vi "UHR-Fleezers Control (fpga) - 11.4b.vi"() -> ()   [LabVIEW 2012]
doc: "UHR-Fleezers Instrument Control Code (fpga)"
uses:
  <vilib>/Platform/TimedLoop/XDataNode/timing_clust.ctl
  <vilib>/Platform/TimedLoop/XDataNode/nitl_modes.ctl
  <vilib>/Platform/TimedLoop/XDataNode/wakeup.ctl
  <vilib>/rvi/eio/common/nirviEmuTemplateMethod_errors.vi
  <vilib>/rvi/interface/RandomDataEmulation/nirviRandomDataFPGAFIFO.vi
  <vilib>/rvi/interface/RandomDataEmulation/niFpgaRandomDataHandleErrors.vi
  <vilib>/rvi/Emulation/niFpgaSctlEmulationGetInTimedLoop.vi
  <vilib>/rvi/Emulation/niFpgaSctlEmulationGlobalWrite.vi
  <vilib>/rvi/Emulation/niFpgaSctlEmulationRegisterWithScheduler.vi
  <vilib>/rvi/Emulation/niFpgaSctlEmulationScheduler.vi
  <vilib>/Platform/TimedLoop/XDataNode/XDataNode.xnode
  <vilib>/eio/EIOMethodNode/EIOMethodNode.xnode
  <vilib>/eio/EIONode/EIONode.xnode
  <vilib>/rvi/DataTransferAndStorage/Container/XNode/niFpgaContainer.xnode
  <vilib>/rvi/interface/RandomDataEmulation/nirviRandomDataFpgaReadWriteTemplate.vi
  <vilib>/addons/control/pid/fpga.llb/XNode/niFpgaPID.xnode
  <vilib>/Platform/TimedLoop/XDataNode/XDNodeRunTimeDep.lvlib
panel:
  in  "Tab Control":T1(tab)=enum."Force FB"
  in  "Set 3":bool
  in  "Set 2":bool=TRUE
  in  "Set 1":bool=TRUE
  in  "Trap Pos to FIFO":bool
  in  "N of AI1 Int Acq Sets":i16=2 min=1 max=3 step=1
  out "AI Late Counter":u8
  in  "ai count":u16=400
  in  "+ phase":bool
  in  "Phase count adjustment":i16
  out "Relative phase":i16
  in  "AI to FIFO":bool
  out "BD1 Frequency Out 1":u64
  out "BD1 Frequency Out 2":u64
  out "Trap Pos FIFO Timeout":u16
  out "Trap AI FIFO Timeout":u16
  in  "Trap FIFO Set Timeout":i32
  in  "Tab Control 2":T2(tab)
  in  "RD":bool
  in  "FB1 output high":i16=3000
  in  "FB1 output low":i16
  in  "D1":i16
  in  "I1":i16=5
  in  "P1":i16=10
  in  "Swap F1 and F2":bool
  in  "Cont. Scan":bool
  in  "Abort scan":bool
  in  "Cycles per step":u64
  in  "Scan BD":bool
  in  "Number of scans":u16
  in  "Scan steps":u64
  in  "Scan freq.  increment":i64
  out "Scanning":bool
  in  "Start scan":bool
  in  "OSK Bd 1":bool
  in  "Reset Bd 1":bool
  in  "PMODE":bool
  in  "Direct RF Box \nCommunication":bool
  in  "Data BD 2":u8 format="%08b"
  in  "Data BD 1":u8 format="%08b"
  in  "Address":u8 format="%02x"
  in  "Update Data":bool
  in  "FPGA Controls\n RF Box":bool
  in  "Number Interlace Cycles":u8=2 min=1 max=3
  in  "Interlace Off Parameters":u8=1 min=1 max=3
  in  "Interlace ON/OFF":bool
  out "DIO Relative phase":i16
  in  "Phase count adjustment (DIO)":i16
  in  "+ phase (DIO)":bool
  out "DIO Late Counter":u8
  in  "DIO count 1 (ticks)":u16=400
  in  "DIO count 2 (ticks)":u16=400
  in  "DIO count 3 (ticks)":u16=400
  out "AI2 Y Sum Set 2":i16
  out "AI2 Y Sum Set 1":i16
  in  "FB Setpoint Set 1":i16 min=0 step=1
  in  "FB Reset Set 1":bool
  in  "FB On/Off Set 1":bool
  in  "FB Reset Set 2":bool
  in  "FB On/Off Set 2":bool
  in  "FB Setpoint Set 2":i16 min=0 step=1
  out "Scan I":u64
  in  "Amp switch delay":u8=5
  in  "BD 2 Amplitude 1":u16
  in  "BD 1 Amplitude 1":u16
  in  "BD 2 Frequency 1":u64
  in  "BD 1 Frequency 1":u64
  in  "BD 2 Amplitude 2":u16
  in  "BD 1 Amplitude 2":u16
  in  "BD 2 Frequency 2":u64
  in  "BD 1 Frequency 2":u64
  in  "BD 2 Amplitude 3":u16
  in  "BD 1 Amplitude 3":u16
  in  "BD 2 Frequency 3":u64
  in  "BD 1 Frequency 3":u64
  in  "BD 1 Delay (ticks)":u8
  in  "BD 2 Delay (Ticks)":u8 caption="Count(Ticks)"
  in  "FB2 output high":fxp<+/-,16,1>=0.999969482421875
  in  "FB2 output low":fxp<+/-,16,1>=-1.0
  in  "P2":fxp<+/-,16,8> format="%.11g"
  in  "I2":fxp<+/-,16,8>=10.0 format="%.11g"
  in  "D2":fxp<+/-,16,8> format="%.11g"
  in  "Negate Diff?":bool
  in  "Diff FB Measurement?":bool
  in  "FB Trig Integrate":u32=1
  out "TTrig?":bool
  in  "TTrig Negate Pos":bool=TRUE
  out "Trap Pos FB Int Signal":fxp<+/-,24,9> format="%.18g"
  out "Trap Pos FB Int-Norm Signal":fxp<+/-,16,1> format="%.16g"
  in  "FPGA TTrig Thresh":i64
  in  "FPGA Trap Trig":bool
  out "Trap Pos FB Action":i64
  in  "Trap Pos. FB Offset Factor":i64
  in  "Trap Pos. FB Mult Factor":i64=2
  in  "Trap Pos. FB Reset":bool
  in  "Trap Pos FB Monitor T1 or T2":bool
  in  "AI1 X Scale":u16
  in  "Trap Pos FB Int Count":u16=100
  in  "Trap Pos FB Negate Action":bool
  out "AI1 X Set 2":fxp<+/-,16,1>
  out "AI1 X Set 1":fxp<+/-,16,1>
  in  "Trap Pos. FB SP":fxp<+/-,16,1>
  in  "Force feedback":bool
  out "TTrig Sig":i64
  out "TTrig Fin Thresh":i64
  in  "1D or 2D Scan?":bool
  in  "Abort scan (MCL)":bool
  in  "MCL Scan Axis":bool
  in  "Cont. Scan (MCL)":bool
  out "Scan I (MCL)":u64
  in  "Number of scans (MCL)":u16
  out "Scanning MCL":bool
  in  "Scan steps (MCL)":u64
  in  "Cycles per step (MCL)":u64
  in  "Scan freq.  increment (MCL)":i16
  in  "Start scan (MCL)":bool
  in  "AO2":i16
  in  "AO1":i16
  out "MCL Late Counter":u8
  in  "MCL count":u32=800
  out "MCL Relative Phase":i16
  in  "Phase count adjustment (MCL)":i16
  in  "+ phase (MCL)":bool
  out "APD3 out state":bool
  in  "APD Gate Operating Mode":u8 max=2 step=1
  in  "Invert APD Gate":bool
  in  "APD Gate OFF Count":u16=100
  in  "APD Gate ON Count":u16=300
  out "APD 1 Gate Late Counter":u8
  out "APD 1 Gate Relative Phase":i16
  in  "Phase count adjustment (APD 1 Gate)":i16
  in  "+ phase (APD 1 Gate)":bool
  out "APD 2 Counts 0":u32
  out "APD 2 Counts 1":u32
  out "APD 1 Counts 0":u32
  out "APD 1 Counts 1":u32
  out "APD1 out state":bool
  in  "APD AO scale factor":i16=1
  in  "APD to FIFO":bool
  in  "APD Acq Rate Count":u32=20000000
  out "APD Acq Late Counter":u8
  out "APD Acq Relative Phase":i16
  in  "Phase Count Adjustment (APD Acq)":i16
  in  "+ phase (APD Acq)":bool
  in  "Phase count adjustment (APD 2 Gate)":i16
  out "APD 2 Gate Late Counter":u8
  out "APD 2 Gate Relative Phase":i16
  in  "+ phase (APD 2 Gate)":bool
  out "APD2 out state":bool
  out "APD 3 Counts 0":u32
  out "APD 3 Counts 1":u32
  out "APD 3 Gate Late Counter":u8
  in  "Phase count adjustment (APD 3 Gate)":i16
  out "APD 3 Gate Relative Phase":i16
  in  "+ phase (APD 3 Gate)":bool
  in  "D3":i16
  in  "I3":i16=5
  in  "P3":i16=10
  in  "Green Filter Flipper":bool
  in  "Green FB Count":u16=1200
  out "Green Late Counter":u8
  out "Green FB Relative Phase":i16
  in  "Phase count adjustment (Green FB)":i16=10
  in  "+ phase (Green FB)":bool
  out "Green FB Sum":i16
  in  "Green int current ON count adj":u16=150
  in  "Current Out":u16=30000
  in  "Green FB On/Off":bool
  in  "Green FB Setpoint":i16=250 min=0 step=1
  in  "Green FB Reset":bool
  in  "Operating Mode 2":u8=2 max=2 step=1
  in  "Invert GI 2":bool
  in  "Green interlace OFF count 2":u16=900
  in  "Green interlace ON count 2":u16=300
  out "GI Late Counter 2":u8
  out "GI Relative phase 2":i16
  in  "Phase count adjustment (GI) 2":i16=20
  in  "+ phase (GI) 2":bool
  in  "Green interlace OFF count":u16=100
  out "GI Relative phase":i16
  in  "Phase count adjustment (GI)":i16
  in  "+ phase (GI)":bool
  in  "Green interlace ON count":u16=300
  out "GI Late Counter":u8
  in  "Invert GI":bool
  in  "Operating Mode":u8 max=2 step=1
  in  "+ phase (RI)":bool
  out "RI Relative phase":i16
  out "RI Late Counter":u8
  in  "Red interlace ON count":u16=300
  in  "Red interlace OFF count":u16=100
  in  "Invert RI":bool
  in  "Red Laser Operating Mode":u8 max=2 step=1
  in  "Phase count adjustment (RI)":i16
  out "Red FB Intensity":i16
  in  "RI Current Out":u16=30000
  in  "Red FB On/Off":bool
  in  "D4":i16
  in  "I4":i16=5
  in  "P4":i16=10
  in  "Red FB Setpoint":i16=250 min=0 step=1
  in  "Red FB Reset":bool
  in  "RI Operating Mode 2":u8=2 max=2 step=1
  in  "Invert RI 2":bool
  in  "Phase count adjustment (BI AO)":i16=20
  in  "Blue current ON count adj (AO)":u16=150
  in  "BI Current Out":i16=30000
  in  "Blue FB On/Off":bool
  in  "D5":i16
  in  "I5":i16=5
  in  "P5":i16=10
  in  "Blue FB Setpoint":i16=250 min=0 step=1
  in  "Blue FB Reset":bool
  in  "BI Operating Mode (AO)":u8=2 max=2 step=1
  in  "Invert BI (AO)":bool
  in  "Blue OFF count (AO)":u16=900
  in  "Blue ON count (AO)":u16=300
  out "BI Late Counter (AO)":u8
  out "BI Relative phase (AO)":i16
  in  "+ phase (BI AO)":bool
  in  "Phase count adjustment (BI D)":i16
  in  "Blue Laser Operating Mode (D)":u8 max=2 step=1
  in  "Invert BI (D)":bool
  in  "Blue interlace OFF count (D)":u16=100
  in  "Blue interlace ON count (D)":u16=300
  out "Blue Late Counter (D)":u8
  out "BI Relative phase (D)":i16
  in  "+ phase (BI D)":bool
  out "Blue Intensity":i16
  # "Only one of these can be on\nat a time:"
  # "Raster Scan AOD"
  # "1 (X)"
  # "2 (Y)"
  # "IR Intensity Feedback (RF BD 1)"
  # "FB Gains Set 1"
  # "FB output range 1"
  # "FB Triggering Excitation Laser"
  # "Trap Pos. FB Gains"
  # "Trap Pos. FB Range"
  # "AO1 (Y)"
  # "2D"
  # "1D"
  # "AO2 (X)"
  # "APD AO for aligning"
  # "Detection Loop"
  # "Green fluorescent laser digital gate interlacing loop"
  # "0 Forced ON\n1 Forced OFF\n2 Interlacing"
  # "Green FB Gains"
  # "Red fluorescent laser digital gate interlacing loop"
  # "Detection Loop"
  # "0 Forced ON\n1 Forced OFF\n2 Interlacing"
  # "Analog/FB Control Loop\n(Disabled)"
  # "Digital Control Loop"
  # "Blue laser intensity reading"
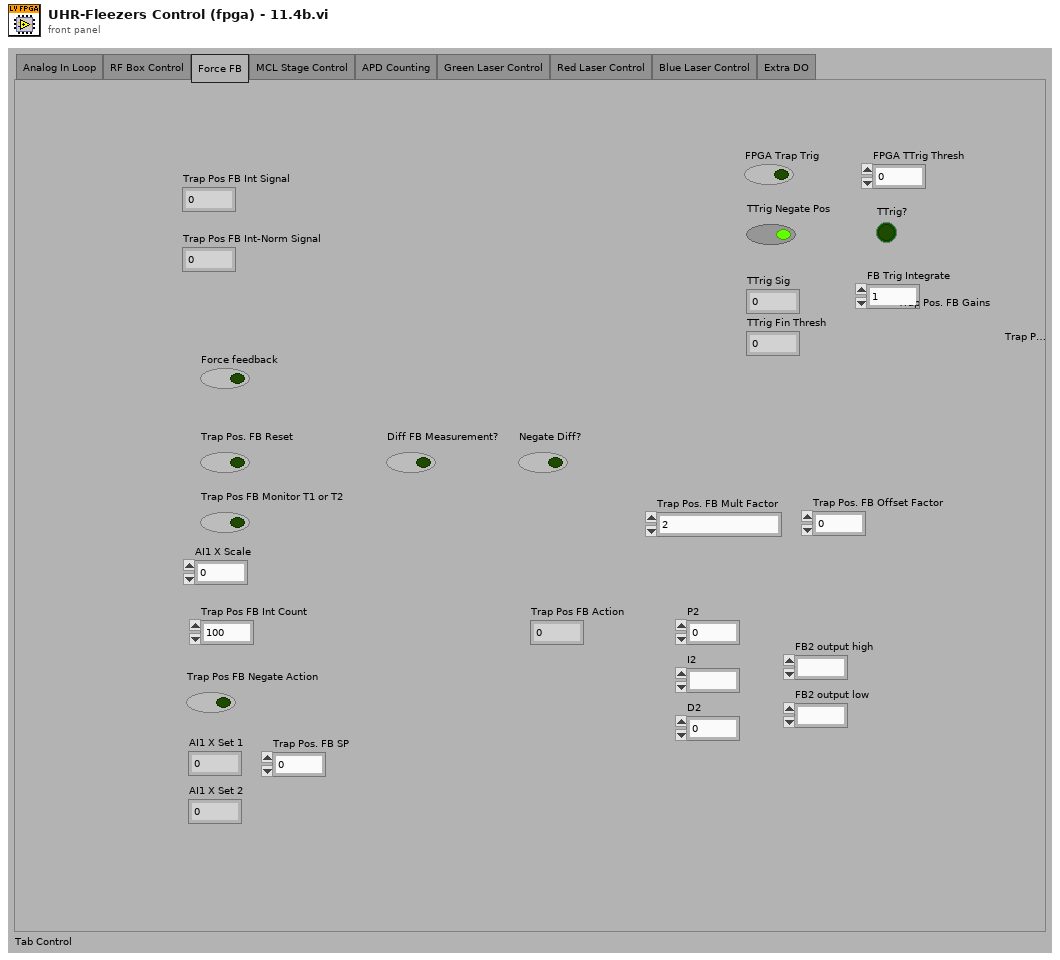
[diagram p1: front panel]
types:
  T1 = enum32{"Analog In Loop", "RF Box Control", "Force FB", "MCL Stage Control", "APD Counting", "Green Laser Control", "Red Laser Control", "Blue Laser Control", "Extra DO"}
  T2 = enum32{"Controls", "Interlacing Frequency and Amplitude Values"}
  T3 = typedef "XDNodeRunTimeDep.lvlib/timing_clust.ctl" = cluster{"Expected End [f-1]":u64, "Actual End [f-1]":u64, "Finished Late? [f-1]":bool, "Expected End [i-1]":u64, "Actual End [i-1]":u64, "Finished Late? [i-1]":bool, "Expected Start [i]":u64, "Actual Start [i]":u64, "Expected Start [f]":u64, "Actual Start [f]":u64, "Source Name":string, "Structure Name":string, "Period":i64, "Deadline":i64, "Offset":i64, "Start":i64, "Priority":i32, "Timeout":i32, "Mode":T4, "Wakeup Reason":T5, "Error":errorcluster, "Source Type":string, "Secondary Source Type":string, "Global End Time":u64, "Global Start Time":u64, "Frame Duration":u64, "Iteration Duration":u64, "Assigned CPU":i32, "I/O Scan Engine Mode":u32}
  T4 = typedef "XDNodeRunTimeDep.lvlib/nitl_modes.ctl" = enum32{"No Change", "Process missed periods, maintain original phase", "Discard missed periods, maintain original phase", "Process missed periods, ignore original phase", "Discard missed periods, ignore original phase"}
  T5 = typedef "XDNodeRunTimeDep.lvlib/wakeup.ctl" = enum32{"Normal", "Aborted", "Asynchronous wakeup", "Timing source error", "Timed loop error", "Timeout"}
  T6 = cluster{"proportional gain (Kc)":i16, "integral gain (Kc*Ts/Ti)":i16, "derivative gain (Kc*Td/Ts)":i16}
  T7 = cluster{"FB1 output high":i16, "FB1 output low":i16}
  T8 = cluster{"P2":fxp<+/-,16,8>, "I2":fxp<+/-,16,8>, "D2":fxp<+/-,16,8>}
  T9 = cluster{"FB2 output high":fxp<+/-,16,1>, "FB2 output low":fxp<+/-,16,1>}
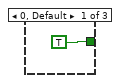
[diagram p3: hidden frame]
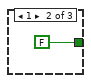
[diagram p4: hidden frame]
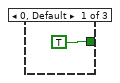
[diagram p5: hidden frame]
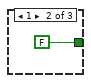
[diagram p6: hidden frame]
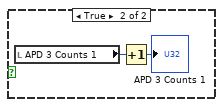
[diagram p7: hidden frame]
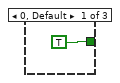
[diagram p8: hidden frame]
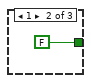
[diagram p9: hidden frame]
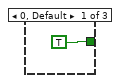
[diagram p10: hidden frame]
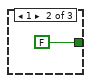
[diagram p11: hidden frame]
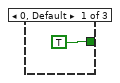
[diagram p12: hidden frame]
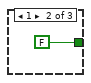
[diagram p13: hidden frame]
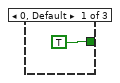
[diagram p14: hidden frame]
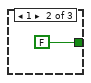
[diagram p15: hidden frame]
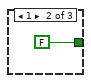
[diagram p18: hidden frame]
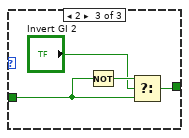
[diagram p19: hidden frame]
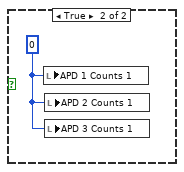
[diagram p20: hidden frame]
diagram:
  w3 = u16 0
  w5 = FALSE
  w2 = FALSE
  # "timing array current index"
  # "timing array"
  # "timing counter (phase adjusted here)"
  # "late counter"
  n1 = flat-sequence "FPGA initialization to do before running any of the loops" {
    tunnel: [u16 0 ("DIO count 3 (ticks)")] -> w1
    tunnel: [w13] -> _
    frame #0 {
      w12 = FALSE ("Enable")
      # "BD 2 (Y)"
      # "BD 1 (X)"
      # "Start up expansion chassis early\nto avoid delays later"
      # "This pin controls udclk on the RF boards.\nWhen initially configuring the boards, this pin needs to be\nconfigured as a high impedance input.  Later it will be switched\nto an output."
      # "Initial setting of DIO data and \naddress to low (before reset).  \nThis needs to happen before the other\ncontrol method loops execute."
      n2 = xnode "FPGA I/O Node"("Chassis2/Mod4/AO0"=u16 0) -> ("Chassis2/Mod1/AI0"=w13:i16)  [unwired: 2 in, 2 out]
      n3 = xnode "FPGA I/O Method Node"("Enable"=w12) -> ()  [unwired: 1 in, 1 out]
      n4 = xnode "FPGA I/O Method Node"("Enable"=w12) -> ()  [unwired: 1 in, 1 out]
      n5 = xnode "FPGA I/O Node"("Connector1/DIO0"=FALSE, "Connector1/DIO1"=FALSE, "Connector1/DIO2"=FALSE, "Connector1/DIO3"=FALSE, "Connector1/DIO4"=FALSE, "Connector1/DIO5"=FALSE, "Connector1/DIO6"=FALSE, "Connector1/DIO7"=FALSE, "Connector1/DIO8"=FALSE, "Connector1/DIO9"=FALSE, "Connector1/DIO10"=FALSE, "Connector1/DIO11"=FALSE, "Connector1/DIO12"=FALSE, "Connector1/DIO13"=FALSE, "Connector1/DIO15"=FALSE, "Connector1/DIO20"=FALSE, "Connector1/DIO21"=FALSE, "Connector1/DIO22"=FALSE, "Connector1/DIO23"=FALSE, "Connector1/DIO24"=FALSE, "Connector1/DIO25"=FALSE, "Connector1/DIO26"=FALSE, "Connector1/DIO27"=FALSE, "Connector1/DIO14"=FALSE) -> ()  [unwired: 24 in, 24 out]
    }
  }
  n6 = local read "AO1"() -> (w10:i16)
  n7 = local read "AO2"() -> (w9:i16)
  n8 = node-c288() -> (w8:T3)  [unwired: 1 in]
  n9 = timed-loop "RF box board DIO control: control bits" {
    timing: w8 -> [_]
    timing-out: [_] -> w7
    tunnel: [w42] -> _
    tunnel: w1 -> [w42]
    stop <- FALSE stop-if-true
    n10 = xnode "FPGA I/O Node"("Connector1/DIO16"="RD", "Connector1/DIO17"="PMODE", "Connector1/DIO18"="OSK Bd 1", "Connector1/DIO19"="Reset Bd 1", "Connector0/DIO3"="Green Filter Flipper") -> ()  [unwired: 5 in, 5 out]
  }
  n11 = while "RF box board DIO control: parallel communication" {
    shift-right: [w55] -> _
    shift-left: w1 -> [w54]
    shift-right: [w53] -> _
    shift-left: FALSE ("Swap F1 and F2") -> [w52]
    stop <- FALSE stop-if-true
    n12 = flat-sequence {
      tunnel: w52 -> [w59]
      tunnel: w54 -> [w57]
      tunnel: [w59] -> w51
      tunnel: [w58] -> w50
      tunnel: [w57] -> w49
      tunnel: [w65] -> w55
      tunnel: [w64] -> w53
      tunnel: w51 -> [w63]
      tunnel: w50 -> [w61]
      tunnel: w49 -> [w60]
      frame #0 {
        n13 = call "Loop Timer"("Count(Ticks)"=w57) -> ("Tick Count(Ticks)"=w58:u16)
      }
      frame #1 {
        n14 = flat-sequence {
          tunnel: ["FPGA Controls\n RF Box"] -> w62
          tunnel: w63 -> [w66]
          tunnel: [w116] -> w65
          tunnel: [w129] -> w64
          tunnel: w62 -> [w128]
          tunnel: w61 -> [w122]
          tunnel: w60 -> [w119]
          frame #0 {
            n15 = case shown="True" "FPGA Controls\n RF Box" {
              tunnel: w66 -> [_ w68]
              frame False {
              }
              frame True {
                n16 = flat-sequence {
                  tunnel: w68 -> [w78]
                  frame #0 {
                    n17 = First Call?() -> (First Call?: T/F=w69:bool)
                    n18 = case shown="True" w69 {
                      frame False {
                      }
                      frame True {
                        # "BD 2"
                        # "BD 1"
                        # "If first time data updated, be sure to set WR high and UDCLK low\nbefore setting data and address bits."
                        n19 = xnode "FPGA I/O Method Node"("Enable"=TRUE) -> ("FPGA I/O Out"=w71:refnum<k21>)  [unwired: 1 in]
                        n20 = xnode "FPGA I/O Method Node"("Enable"=TRUE) -> ("FPGA I/O Out"=w74:refnum<k21>)  [unwired: 1 in]
                        n21 = xnode "FPGA I/O Node"("Connector1/DIO15"=TRUE) -> ()  [unwired: 1 in, 1 out]
                        n22 = xnode "FPGA I/O Node"("I/O Item"=FALSE ("Connector1/DIO30"), "FPGA I/O In"=w71) -> ()  [unwired: 1 out]
                        n23 = xnode "FPGA I/O Node"("I/O Item"=FALSE ("Connector1/DIO30"), "FPGA I/O In"=w74) -> ()  [unwired: 1 out]
                      }
                    }
                  }
                  frame #1 {
                    n24 = flat-sequence "BD 1 (X)" {
                      tunnel: w78 -> [w85]
                      tunnel: "Amp switch delay" -> [w86]
                      frame #0 {
                        n25 = call "Wait6"("Count(Ticks)"="BD 1 Delay (ticks)") -> ()  [unwired: 1 out]
                      }
                      frame #1 {
                        # "switch frequency"
                        n26 = xnode "FPGA I/O Node"("Connector1/DIO36"=w85) -> ()  [unwired: 1 in, 1 out]
                      }
                      frame #2 {
                        # "~5 ticks is usual"
                        n27 = call "Wait4"("Count(Ticks)"=w86) -> ()  [unwired: 1 out]
                      }
                      frame #3 {
                        # "this switches amplitude"
                        # "switch amplitude"
                        # "send udclk high"
                        n28 = xnode "FPGA I/O Node"("Connector1/DIO30"=TRUE ("Connector1/DIO15")) -> ()  [unwired: 1 in, 1 out]
                      }
                      frame #4 {
                        # "reset to be ready for next\ncycle"
                        # "send udclk low"
                        n29 = xnode "FPGA I/O Node"("Connector1/DIO30"=FALSE ("Connector1/DIO15")) -> ()  [unwired: 1 in, 1 out]
                      }
                    }
                    n30 = flat-sequence "BD 2 (Y)" {
                      tunnel: w78 -> [w80]
                      tunnel: "Amp switch delay" -> [w81]
                      frame #0 {
                        n31 = call "Wait7"("Count(Ticks)"="BD 2 Delay (Ticks)") -> ()  [unwired: 1 out]
                      }
                      frame #1 {
                        # "switch frequency"
                        n32 = xnode "FPGA I/O Node"("Connector1/DIO37"=w80) -> ()  [unwired: 1 in, 1 out]
                      }
                      frame #2 {
                        # "~5 ticks is usual"
                        n33 = call "Wait5"("Count(Ticks)"=w81) -> ()  [unwired: 1 out]
                      }
                      frame #3 {
                        # "this switches amplitude"
                        # "switch amplitude"
                        # "send udclk high"
                        n34 = xnode "FPGA I/O Node"("Connector1/DIO29"=TRUE ("Connector1/DIO15")) -> ()  [unwired: 1 in, 1 out]
                      }
                      frame #4 {
                        # "reset to be ready for next\ncycle"
                        # "send udclk low"
                        n35 = xnode "FPGA I/O Node"("Connector1/DIO29"=FALSE ("Connector1/DIO15")) -> ()  [unwired: 1 in, 1 out]
                      }
                    }
                  }
                }
              }
            }
          }
          frame #1 {
            # "This is the prior cycle's on time"
            # "increment timing\nindex, reset to 0 if \nend of matrix"
            # "Reset to begginning (1) when number of cycles reached."
            # "timing index"
            # "build byte stacks for writing data\n(must correspond to addresses array constant)"
            # "Timing housekeeping"
            # "Adjust phase if late\n(maintains constant phase relationship between cycles)"
            n36 = Bundle("FB1 output high"="FB1 output high", "FB1 output low"="FB1 output low") -> (w89:T7)  [unwired: 1 in]
            n37 = Bundle("P1"="P1", "I1"="I1", "D1"="D1") -> (w90:cluster{"P1":i16, "I1":i16, "D1":i16})  [unwired: 1 in]
            n38 = feedback #1(u8 0 ("t")) -> (w125:u8)
            n39 = Increment(x=w125) -> (x+1=w169:u8)
            n40 = Increment(x="Number Interlace Cycles") -> (x+1=w164:u8)
            n41 = Equal?(x=w169, y=w164) -> (x = y?=w171:bool)
            n42 = Select(t=u8 1, s=w171, f=w169) -> (s? t:f=w124:u8)
            n43 = feedback-in #1(w124) -> ()
            n44 = Increment(x=w124) -> (x+1=w166:u8)
            n45 = Equal?(x=w166, y=w164) -> (x = y?=w167:bool)
            n46 = Select(t=u8 1, s=w167, f=w166) -> (s? t:f=w163:u8)
            n47 = Select(t=w163, s="Interlace ON/OFF", f="Interlace Off Parameters") -> (s? t:f=w147:u8)
            n48 = case shown="1, Default" w147 {
              tunnel: [w243 "BD 1 Frequency 2" "BD 1 Frequency 3"] -> w159
              tunnel: [w242 "BD 2 Frequency 2" "BD 2 Frequency 3"] -> w148
              tunnel: ["BD 2 Amplitude 1" "BD 2 Amplitude 2" "BD 2 Amplitude 3"] -> w104
              tunnel: [w231 w402 "BD 1 Amplitude 3"] -> w107
              tunnel: w90 -> [w205 w399 _]
              tunnel: w89 -> [w206 w398 _]
              frame 1, Default {
                w222 = fxp<+/-,24,9> 0.0 ("AI1 X Set 2")
                w215 = u16 0
                w238 = u64 0 ("f")
                # "This signal integration happens no matter what\nso that correct setpoints can be chosen before \nturning on the FB."
                # "Trap 1"
                n49 = local read "AI1 X Set 2"() -> (w218:fxp<+/-,16,1>)
                n50 = local read "AI1 X Set 1"() -> (w219:fxp<+/-,16,1>)
                n51 = local read "Scanning"() -> (w244:bool)
                n52 = Or(x=w244, y="Start scan") -> (x .or. y?=w236:bool)
                n53 = case shown="False" "Diff FB Measurement?" {
                  tunnel: w218 -> [w252 w261]
                  tunnel: w219 -> [w251 w262]
                  tunnel: [w249 w253] -> w220
                  frame False {
                    n54 = Select(t=w251, s="Trap Pos FB Monitor T1 or T2", f=w252) -> (s? t:f=w249:fxp<+/-,16,1>)
                  }
                  frame True {
                    n55 = Subtract(x=w262, y=w261) -> (x-y=w254:fxp<+/-,17,2>)
                    n56 = Not(x="Negate Diff?") -> (.not. x?=w260:bool)
                    n57 = Boolean To (0,1)(Boolean="Negate Diff?") -> (0, 1=w258:i16)
                    n58 = Boolean To (0,1)(Boolean=w260) -> (0, 1=w259:i16)
                    n59 = Negate(x=w258) -> (-x=w257:i16)
                    n60 = Add(x=w257, y=w259) -> (x+y=w255:i16)
                    n61 = Multiply(x=w255, y=w254) -> (x*y=w253:fxp<+/-,32,17>)
                  }
                }
                n62 = Not(x="Abort scan") -> (.not. x?=w234:bool)
                n63 = And(x=w234, y=w236) -> (x .and. y?=w233:bool)
                n64 = case "For raster scanning" shown="True" w233 {
                  tunnel: [u64 0 w388] -> w239
                  tunnel: "Start scan" -> [_ w373]
                  frame False {
                    n65 = local write "Scanning"(FALSE ("scanning")) -> ()
                  }
                  frame True {
                    w357 = i64 0
                    w356 = u64 0
                    # "scan incr."
                    # "freq. incr. mult."
                    # "count steps"
                    # "count number of cycles"
                    n66 = feedback #2(w356) -> (w385:u64)
                    n67 = Select(t=w356, s=w373, f=w385) -> (s? t:f=w387:u64)
                    n68 = Increment(x=w387) -> (x+1=w384:u64)
                    n69 = Greater?(x="Cycles per step", y=w384) -> (0:w366:bool)
                    n70 = Select(t=w384, s=w366, f=w356) -> (s? t:f=w383:u64)
                    n71 = feedback-in #2(w383) -> ()
                    n72 = feedback #3(w356) -> (w382:u64)
                    n73 = Select(t=w356, s=w373, f=w382) -> (s? t:f=w377:u64)
                    n74 = Increment(x=w377) -> (x+1=w381:u64)
                    n75 = Add(x="Scan steps", y="Scan steps") -> (x+y=w380:u64)
                    n76 = Select(t=w377, s=w366, f=w381) -> (s? t:f=w361:u64)
                    n77 = Greater?(x=w380, y=w361) -> (0:w360:bool)
                    n78 = Select(t=w361, s=w360, f=w356) -> (s? t:f=w378:u64)
                    n79 = feedback-in #3(w378) -> ()
                    n80 = Equal?(x="Scan steps", y=w361) -> (x = y?=w365:bool)
                    n81 = Greater?(x="Scan steps", y=w377) -> (0:w376:bool)
                    n82 = feedback #4(w357) -> (w379:i64)
                    n83 = Select(t=w357, s=w373, f=w379) -> (s? t:f=w363:i64)
                    n84 = Increment(x=w363) -> (x+1=w375:i64)
                    n85 = Decrement(x=w363) -> (x-1=w374:i64)
                    n86 = Select(t=w375, s=w376, f=w374) -> (s? t:f=w364:i64)
                    n87 = Select(t=w363, s=w365, f=w364) -> (s? t:f=w362:i64)
                    n88 = Select(t=w363, s=w366, f=w362) -> (s? t:f=w358:i64)
                    n89 = Select(t=w358, s=w360, f=w357) -> (s? t:f=w359:i64)
                    n90 = feedback-in #4(w359) -> ()
                    n91 = feedback #5(w356) -> (w372:u64)
                    n92 = Select(t=w356, s=w373, f=w372) -> (s? t:f=w368:u64)
                    n93 = Increment(x=w368) -> (x+1=w369:u64)
                    n94 = Select(t=w368, s=w360, f=w369) -> (s? t:f=w367:u64)
                    n95 = Greater?(x="Number of scans", y=w367) -> (0:w353:bool)
                    n96 = Multiply(x="Scan freq.  increment", y=w363) -> (x*y=w388:i64)
                    n97 = Select(t=TRUE, s="Cont. Scan", f=w353) -> (s? t:f=w352:bool)
                    "Scanning" <- w352
                    n98 = Select(t=w367, s=w352, f=w356) -> (s? t:f=w370:u64)
                    n99 = feedback-in #5(w370) -> ()
                    n100 = Increment(x=w367) -> (x+1=→"Scan I":u64)
                  }
                }
                n101 = feedback #6(w215) -> (w214:u16)
                n102 = Increment(x=w214) -> (x+1=w216:u16)
                n103 = Greater Or Equal?(x=w216, y="Trap Pos FB Int Count") -> (x >= y?=w207:bool)
                n104 = Select(t=w215, s=w207, f=w216) -> (s? t:f=w217:u16)
                n105 = feedback-in #6(w217) -> ()
                n106 = feedback #7(w222) -> (w221:fxp<+/-,24,9>)
                n107 = Add(x=w220, y=w221) -> (x+y=w213:fxp<+/-,24,9>)
                n108 = case "For intensity feedback" shown="True" "FB On/Off Set 1" {
                  tunnel: "BD 1 Amplitude 1" -> [w390 _]
                  tunnel: [w390 w394] -> w231
                  tunnel: w206 -> [_ w391]
                  tunnel: w205 -> [_ w392]
                  frame False {
                  }
                  frame True {
                    n109 = local read "AI2 Y Sum Set 1"() -> (w395:i16)
                    n110 = call "Slower PID.vi"("process variable"=w395, "reset?"="FB Reset Set 1", "setpoint"="FB Setpoint Set 1", "PID gains (x 2^8)"=w392, "output range"=w391) -> ("output"=w396:i16)  [unwired: 10 out]
                    n111 = To Unsigned Word Integer(number=w396) -> (unsigned 16bit integer=w394:u16)
                  }
                }
                n112 = Select(t=w222, s=w207, f=w213) -> (s? t:f=w225:fxp<+/-,24,9>)
                n113 = feedback-in #7(w225) -> ()
                n114 = Divide(x=w213, y="Trap Pos FB Int Count") -> (x/y=w208:fxp<+/-,16,1>)
                n115 = feedback #8(fxp<+/-,24,9> 0.0 ("AI1 X Set 2")) -> (w226:fxp<+/-,24,9>)
                n116 = Select(t=w213, s=w207, f=w226) -> (s? t:f=w227:fxp<+/-,24,9>)
                "Trap Pos FB Int Signal" <- w227
                n117 = feedback-in #8(w227) -> ()
                n118 = feedback #9(fxp<+/-,16,1> 0.0 ("Trap Pos FB Int-Norm Signal")) -> (w210:fxp<+/-,16,1>)
                n119 = Select(t=w208, s=w207, f=w210) -> (s? t:f=w209:fxp<+/-,16,1>)
                "Trap Pos FB Int-Norm Signal" <- w209
                n120 = feedback-in #9(w209) -> ()
                n121 = case "For position feedback" shown="True" "Force feedback" {
                  tunnel: [i64 0 w268] -> w228
                  tunnel: w208 -> [_ w265]
                  tunnel: w207 -> [_ w264]
                  frame False {
                  }
                  frame True {
                    n122 = feedback #10(i64 0) -> (w267:i64)
                    n123 = case shown="True" w264 {
                      tunnel: [w269 w283] -> w268
                      tunnel: w267 -> [w269 _]
                      tunnel: w265 -> [_ w277]
                      frame False {
                      }
                      frame True {
                        w287 = u32 0
                        n124 = Bundle("P2"="P2", "I2"="I2", "D2"="D2") -> (w273:T8)  [unwired: 1 in]
                        n125 = Bundle("FB2 output high"="FB2 output high", "FB2 output low"="FB2 output low") -> (w270:T9)  [unwired: 1 in]
                        n126 = xnode ("PID")("process variable"=w277, "reset?"="Trap Pos. FB Reset", "setpoint"="Trap Pos. FB SP", "PID gains"=w273, "output range"=w270) -> ("output"=w299:fxp<+/-,16,1>)
                        n127 = Negate(x=w299) -> (-x=w298:fxp<+/-,17,2>)
                        n128 = Select(t=w298, s="Trap Pos FB Negate Action", f=w299) -> (s? t:f=w295:fxp<+/-,17,2>)
                        n129 = Scale By Power Of 2(n=u32 15, x=u32 1) -> (x*2^n=w292:u32)
                        n130 = Multiply(x=w295, y=w292) -> (x*y=w291:fxp<+/-,17,17>)
                        n131 = To Quad Integer(1:w291) -> (0:w303:i64)
                        "Trap Pos FB Action" <- w303
                        n132 = Multiply(x=w303, y="Trap Pos. FB Mult Factor") -> (x*y=w301:i64)
                        n133 = Add(x=w301, y="Trap Pos. FB Offset Factor") -> (x+y=w283:i64)
                        n134 = feedback #11() -> (w284:i64)  [unwired: 1 in]
                        n135 = Add(x=w283, y=w284) -> (x+y=w281:i64)
                        n136 = feedback #12(w287) -> (w289:u32)
                        n137 = Increment(x=w289) -> (x+1=w278:u32)
                        n138 = Greater Or Equal?(x=w278, y="FB Trig Integrate") -> (x >= y?=w279:bool)
                        n139 = Select(t=i64 0, s=w279, f=w281) -> (s? t:f=w285:i64)
                        n140 = feedback-in #11(w285) -> ()
                        n141 = Select(t=w287, s=w279, f=w278) -> (s? t:f=w288:u32)
                        n142 = feedback-in #12(w288) -> ()
                        n143 = And(x=w279, y="FPGA Trap Trig") -> (x .and. y?=w286:bool)
                        n144 = case "Trap FB trigger excitation laser ON" shown="True" w286 {
                          tunnel: w281 -> [_ w307]
                          tunnel: w278 -> [_ w305]
                          frame False {
                          }
                          frame True {
                            n145 = Not(x="TTrig Negate Pos") -> (.not. x?=w314:bool)
                            n146 = Boolean To (0,1)(Boolean="TTrig Negate Pos") -> (0, 1=w312:i16)
                            n147 = Boolean To (0,1)(Boolean=w314) -> (0, 1=w313:i16)
                            n148 = Negate(x=w312) -> (-x=w311:i16)
                            n149 = Add(x=w311, y=w313) -> (x+y=w310:i16)
                            n150 = Multiply(x=w310, y=w307) -> (x*y=w309:i64)
                            "TTrig Sig" <- w309
                            n151 = Multiply(x="FPGA TTrig Thresh", y=w305) -> (x*y=w306:i64)
                            "TTrig Fin Thresh" <- w306
                            n152 = Greater Or Equal?(x=w309, y=w306) -> (x >= y?=w308:bool)
                            n153 = case shown="True" w308 {
                              frame False {
                              }
                              frame True {
                                w317 = TRUE ("Green FB On/Off")
                                w319 = u8 2 ("Operating Mode")
                                n154 = local write "Operating Mode 2"(w319) -> ()
                                n155 = local write "Operating Mode"(w319) -> ()
                                n156 = local write "Green FB On/Off"(w317) -> ()
                                n157 = local write "FPGA Trap Trig"(FALSE ("FPGA Trap Trig")) -> ()
                                "TTrig?" <- w317
                              }
                            }
                          }
                        }
                      }
                    }
                    n158 = feedback-in #10(w268) -> ()
                  }
                }
                n159 = Select(t=w238, s="Scan BD", f=w239) -> (s? t:f=w237:u64)
                n160 = Select(t=w239, s="Scan BD", f=w238) -> (s? t:f=w240:u64)
                n161 = Add(x=w237, y="BD 2 Frequency 1") -> (x+y=w242:u64)
                n162 = Compound Arithmetic op=ADD("BD 1 Frequency 1", w228, w240) -> (w243:u64)
                "BD1 Frequency Out 1" <- w243
              }
              frame 2 {
                # "Trap 2"
                n163 = case shown="True" "FB On/Off Set 2" {
                  tunnel: [w406 w409] -> w402
                  tunnel: "BD 1 Amplitude 2" -> [w406 _]
                  tunnel: w399 -> [_ w408]
                  tunnel: w398 -> [_ w407]
                  frame False {
                  }
                  frame True {
                    n164 = local read "AI2 Y Sum Set 2"() -> (w412:i16)
                    n165 = call "Slower PID.vi"("process variable"=w412, "reset?"="FB Reset Set 2", "setpoint"="FB Setpoint Set 2", "PID gains (x 2^8)"=w408, "output range"=w407) -> ("output"=w410:i16)  [unwired: 10 out]
                    n166 = To Unsigned Word Integer(number=w410) -> (unsigned 16bit integer=w409:u16)
                  }
                }
                "BD1 Frequency Out 2" <- "BD 1 Frequency 2"
              }
              frame 3 {
                # "Fluorescence period"
              }
            }
            n167 = feedback-in #13(w122) -> ()
            n168 = feedback #13(w122) -> (w121:u16)
            n169 = Select(t=w124, s="Interlace ON/OFF", f="Interlace Off Parameters") -> (s? t:f=w162:u8)
            n170 = Subtract(x=w122, y=w121) -> (x-y=w120:u16)
            n171 = Subtract "The error"(x=w120, y=w119) -> (x-y=w97:u16)
            n172 = case shown="1, Default" w162 {
              tunnel: ["DIO count 1 (ticks)" "DIO count 2 (ticks)" "DIO count 3 (ticks)"] -> w118
              frame 1, Default {
              }
              frame 2 {
              }
              frame 3 {
              }
            }
            n173 = Number To Boolean Array(number=w97) -> (Boolean array=w98:bool[])
            n174 = Or Array Elements(Boolean array=w98) -> (logical OR=w96:bool)
            n175 = Boolean To (0,1)(Boolean=w96) -> (0, 1=w103:i16)
            n176 = To Unsigned Byte Integer(number=w103) -> (unsigned 8bit integer=w100:u8)
            n177 = feedback #14(u8 0) -> (w101:u8)
            n178 = Add(x=w100, y=w101) -> (x+y=w99:u8)
            "DIO Late Counter" <- w99
            n179 = feedback-in #14(w99) -> ()
            n180 = Subtract(x=w118, y=w97) -> (x-y=w117:u16)
            n181 = Split Number(x=w159) -> (hi(x)=w158:u32, lo(x)=w157:u32)
            n182 = Split Number(x=w148) -> (hi(x)=w153:u32, lo(x)=w152:u32)
            n183 = Boolean To (0,1)(Boolean="+ phase (DIO)") -> (0, 1=w114:i16)
            n184 = Split Number(x=w158) -> (lo(x)=w156:u16)  [unwired: 1 out]
            n185 = Split Number(x=w157) -> (hi(x)=w155:u16, lo(x)=w154:u16)
            n186 = Split Number(x=w153) -> (lo(x)=w151:u16)  [unwired: 1 out]
            n187 = Split Number(x=w152) -> (hi(x)=w150:u16, lo(x)=w149:u16)
            n188 = Split Number(x=w107) -> (hi(x)=w109:u8, lo(x)=w108:u8)
            n189 = Split Number(x=w104) -> (hi(x)=w106:u8, lo(x)=w105:u8)
            n190 = Split Number(x=w156) -> (hi(x)=w146:u8, lo(x)=w145:u8)
            n191 = Split Number(x=w155) -> (hi(x)=w144:u8, lo(x)=w143:u8)
            n192 = Split Number(x=w151) -> (hi(x)=w139:u8, lo(x)=w138:u8)
            n193 = Split Number(x=w154) -> (hi(x)=w142:u8, lo(x)=w141:u8)
            n194 = Split Number(x=w150) -> (hi(x)=w137:u8, lo(x)=w136:u8)
            n195 = Split Number(x=w149) -> (hi(x)=w135:u8, lo(x)=w134:u8)
            n196 = Multiply(x=w114, y="Phase count adjustment (DIO)") -> (x*y=w110:i16)
            n197 = feedback #15(i16 0) -> (w112:i16)
            n198 = Subtract(x=w112, y=w110) -> (x-y=w111:i16)
            "DIO Relative phase" <- w111
            n199 = feedback-in #15(w111) -> ()
            n200 = Add(x=w117, y=w110) -> (x+y=w116:u16)
            n201 = Build Array "BD 1 A Stack"(w109, w108) -> (w131:u8[])
            n202 = Build Array "BD 2 A Stack"(w106, w105) -> (w130:u8[])
            n203 = Build Array "BD 1 nu Stack"(w146, w145, w144, w143, w142, w141) -> (w140:u8[])
            n204 = Build Array "BD 2 nu Stack"(w139, w138, w137, w136, w135, w134) -> (w133:u8[])
            n205 = case shown="2" w147 {
              tunnel: [w197 w200] -> w129
              tunnel: [u8 10 u8 4] -> w132
              tunnel: "Swap F1 and F2" -> [w198 w200]
              frame 2 {
                # "F2"
                n206 = Not(x=w198) -> (.not. x?=w197:bool)
              }
              frame 1, Default {
                # "low chooses F1"
                # "F1"
              }
            }
            n207 = case "If FPGA is controlling (toggling) RF synth" shown="True" w128 {
              tunnel: w140 -> [_ w176]
              tunnel: w133 -> [_ w175]
              tunnel: w132 -> [_ w174]
              tunnel: w131 -> [_ w173]
              tunnel: w130 -> [_ w172]
              frame False {
              }
              frame True {
                # "Write next amp.\n(wait until beginning of next loop iteration to update)"
                n208 = flat-sequence "Update the next F1 and F2 frequency value (the actual frequency won't change until FSK is switched).\nThen load the next amplitude value into buffer, but don't update it until the next cycle." {
                  tunnel: w176 -> [w179]
                  tunnel: w175 -> [w178]
                  tunnel: w174 -> [w177]
                  tunnel: w173 -> [w190]
                  tunnel: w172 -> [w189]
                  frame #0 {
                    n209 = for {
                      tunnel: w179 -> [w185] mode=indexing
                      tunnel: w178 -> [w184] mode=indexing
                      tunnel: w177 -> [w182]
                      i -> [w183]
                      # "Write next freq."
                      n210 = To Unsigned Byte Integer(number=w183) -> (unsigned 8bit integer=w180:u8)
                      n211 = Add(x=w182, y=w180) -> (x+y=w181:u8)
                      n212 = call "write to RF synth bd.vi"("Address Byte"=w181, "BD 2 Byte"=w184, "BD 1 Byte"=w185) -> ()
                    }
                  }
                  frame #1 {
                    w186 = TRUE ("Connector1/DIO15")
                    # "send udclk high\n(BD 1 and 2)"
                    n213 = xnode "FPGA I/O Node"("Connector1/DIO30"=w186, "Connector1/DIO29"=w186) -> ()  [unwired: 2 in, 2 out]
                  }
                  frame #2 {
                    w187 = FALSE ("Connector1/DIO15")
                    n214 = xnode "FPGA I/O Node"("Connector1/DIO30"=w187, "Connector1/DIO29"=w187) -> ()  [unwired: 2 in, 2 out]
                  }
                  frame #3 {
                    n215 = for {
                      tunnel: w190 -> [w196] mode=indexing
                      tunnel: w189 -> [w195] mode=indexing
                      tunnel: u8 33 -> [w193]
                      i -> [w194]
                      n216 = To Unsigned Byte Integer(number=w194) -> (unsigned 8bit integer=w191:u8)
                      n217 = Add(x=w193, y=w191) -> (x+y=w192:u8)
                      n218 = call "write to RF synth bd.vi"("Address Byte"=w192, "BD 2 Byte"=w195, "BD 1 Byte"=w196) -> ()
                    }
                  }
                }
              }
            }
          }
        }
      }
    }
  }
  n219 = while "RF box board direct communication loop" {
    tunnel: w1 -> [_]
    stop <- FALSE stop-if-true
    n220 = case "Whether to use direct communication method (only use one method at a time)" shown="True" "Direct RF Box \nCommunication" {
      frame False {
      }
      frame True {
        n221 = case shown="True" "Update Data" {
          frame False {
          }
          frame True {
            n222 = flat-sequence {
              frame #0 {
                n223 = First Call?() -> (First Call?: T/F=w421:bool)
                n224 = case shown="True" w421 {
                  frame False {
                  }
                  frame True {
                    # "If first time data updated, be sure to set WR high\nbefore setting data and address bits."
                    n225 = flat-sequence {
                      frame #0 {
                        n226 = xnode "FPGA I/O Node"("Connector1/DIO15"=TRUE) -> ()  [unwired: 1 in, 1 out]
                      }
                      frame #1 {
                        n227 = call "Wait"("Count(Ticks)"=u8 40 ("DO Delay 3 (Ticks)")) -> ()  [unwired: 1 out]
                      }
                    }
                  }
                }
              }
              frame #1 {
                n228 = Number To Boolean Array(number="Address") -> (Boolean array=w470:bool[])
                n229 = Number To Boolean Array(number="Data BD 1") -> (Boolean array=w471:bool[])
                n230 = Number To Boolean Array(number="Data BD 2") -> (Boolean array=w440:bool[])
                n231 = Index Array(array=w471, index=7) -> (element=w455:bool)
                n232 = Index Array(array=w471, index=6) -> (element=w454:bool)
                n233 = Index Array(array=w471, index=5) -> (element=w453:bool)
                n234 = Index Array(array=w471, index=4) -> (element=w452:bool)
                n235 = Index Array(array=w471, index=3) -> (element=w451:bool)
                n236 = Index Array(array=w471, index=2) -> (element=w450:bool)
                n237 = Index Array(array=w471, index=1) -> (element=w449:bool)
                n238 = Index Array(array=w471, index=0) -> (element=w448:bool)
                n239 = Index Array(array=w470, index=5) -> (element=w447:bool)
                n240 = Index Array(array=w470, index=4) -> (element=w446:bool)
                n241 = Index Array(array=w470, index=3) -> (element=w445:bool)
                n242 = Index Array(array=w470, index=2) -> (element=w444:bool)
                n243 = Index Array(array=w470, index=1) -> (element=w443:bool)
                n244 = Index Array(array=w470, index=0) -> (element=w442:bool)
                n245 = Index Array(array=w440, index=7) -> (element=w431:bool)
                n246 = Index Array(array=w440, index=6) -> (element=w430:bool)
                n247 = Index Array(array=w440, index=5) -> (element=w429:bool)
                n248 = Index Array(array=w440, index=4) -> (element=w428:bool)
                n249 = Index Array(array=w440, index=3) -> (element=w427:bool)
                n250 = Index Array(array=w440, index=2) -> (element=w426:bool)
                n251 = Index Array(array=w440, index=1) -> (element=w425:bool)
                n252 = Index Array(array=w440, index=0) -> (element=w424:bool)
                n253 = xnode "FPGA I/O Node"("Connector1/DIO0"=w455, "Connector1/DIO1"=w454, "Connector1/DIO2"=w453, "Connector1/DIO3"=w452, "Connector1/DIO4"=w451, "Connector1/DIO5"=w450, "Connector1/DIO6"=w449, "Connector1/DIO7"=w448, "Connector1/DIO8"=w447, "Connector1/DIO9"=w446, "Connector1/DIO10"=w445, "Connector1/DIO11"=w444, "Connector1/DIO12"=w443, "Connector1/DIO13"=w442, "Connector1/DIO20"=w431, "Connector1/DIO21"=w430, "Connector1/DIO22"=w429, "Connector1/DIO23"=w428, "Connector1/DIO24"=w427, "Connector1/DIO25"=w426, "Connector1/DIO26"=w425, "Connector1/DIO27"=w424) -> ()  [unwired: 22 in, 22 out]
              }
              frame #2 {
                # "wait and then apply write signal"
                n254 = call "Wait2"("Count(Ticks)"=u8 40 ("DO Delay 1 (Ticks)")) -> ()  [unwired: 1 out]
              }
              frame #3 {
                # "sending bit low writes data to board buffer"
                n255 = xnode "FPGA I/O Node"("Connector1/DIO15"=FALSE) -> ()  [unwired: 1 in, 1 out]
              }
              frame #4 {
                # "wait then return write signal"
                n256 = call "Wait3"("Count(Ticks)"=u8 40 ("DO Delay 2 (Ticks)")) -> ()  [unwired: 1 out]
              }
              frame #5 {
                # "sending bit high makes ready to\nwrite more data"
                n257 = xnode "FPGA I/O Node"("Connector1/DIO15"=TRUE) -> ()  [unwired: 1 in, 1 out]
              }
            }
          }
        }
      }
    }
  }
  n258 = To Unsigned Long Integer(number=w1) -> (unsigned 32bit integer=w6:u32)
  n259 = while "APD 1 Counter" {
    tunnel: w1 -> [_]
    stop <- FALSE stop-if-true
    n260 = flat-sequence {
      frame #0 {
        n261 = xnode "FPGA I/O Method Node"("FPGA I/O In"=refnum<k21> "Connector0/DIO0" ("APD 1 DO"), "Timeout"=-1) -> ()  [unwired: 2 out]
      }
      frame #1 {
        n262 = local read "APD1 out state"() -> (w481:bool)
        n263 = case shown="False" w481 {
          frame False {
            n264 = local read "APD 1 Counts 0"() -> (w483:u32)
            n265 = Increment(x=w483) -> (x+1=→"APD 1 Counts 0":u32)
          }
          frame True {
            n266 = local read "APD 1 Counts 1"() -> (w485:u32)
            n267 = Increment(x=w485) -> (x+1=→"APD 1 Counts 1":u32)
          }
        }
      }
    }
  }
  n268 = while "APD 2 Counter" {
    tunnel: w1 -> [_]
    stop <- FALSE stop-if-true
    n269 = flat-sequence {
      frame #0 {
        n270 = xnode "FPGA I/O Method Node"("FPGA I/O In"=refnum<k21> "Connector0/DIO1" ("APD 2 DO"), "Timeout"=-1) -> ()  [unwired: 2 out]
      }
      frame #1 {
        n271 = local read "APD2 out state"() -> (w489:bool)
        n272 = case shown="False" w489 {
          frame False {
            n273 = local read "APD 2 Counts 0"() -> (w491:u32)
            n274 = Increment(x=w491) -> (x+1=→"APD 2 Counts 0":u32)
          }
          frame True {
            n275 = local read "APD 2 Counts 1"() -> (w493:u32)
            n276 = Increment(x=w493) -> (x+1=→"APD 2 Counts 1":u32)
          }
        }
      }
    }
  }
  n277 = while "APD 2 Gating" {
    shift-right: [w497] -> _
    shift-left: w1 -> [w502]
    shift-right: [w496] -> _
    shift-left: w5 -> [w494]
    stop <- FALSE stop-if-true
    n278 = flat-sequence {
      tunnel: w502 -> [w505]
      tunnel: [w506] -> w500
      tunnel: [w505] -> w498
      tunnel: [w504] -> w495
      tunnel: w494 -> [w504]
      tunnel: [w509] -> w501
      tunnel: w500 -> [w509]
      tunnel: [w508] -> w499
      tunnel: w498 -> [w508]
      tunnel: w495 -> [w507]
      tunnel: [w527] -> w497
      tunnel: w501 -> [w538]
      tunnel: w499 -> [w536]
      tunnel: [w531] -> w496
      frame #0 {
        n279 = call "Loop Timer8"("Count(Ticks)"=w505) -> ("Tick Count(Ticks)"=w506:u16)
      }
      frame #1 {
        # "Signal is then sent through \na transistor before APD"
        n280 = xnode "FPGA I/O Node"("Connector0/DIO8"=w507) -> ()  [unwired: 1 in, 1 out]
      }
      frame #2 {
        n281 = local read "APD Gate ON Count"() -> (w520:u16)
        n282 = local read "APD Gate OFF Count"() -> (w519:u16)
        n283 = feedback #16(TRUE) -> (w533:bool)
        n284 = feedback-in #17(w538) -> ()
        n285 = feedback #17(w538) -> (w521:u16)
        n286 = Not(x=w533) -> (.not. x?=w530:bool)
        n287 = feedback-in #16(w530) -> ()
        n288 = Subtract(x=w538, y=w521) -> (x-y=w537:u16)
        n289 = Select(t=w520, s=w530, f=w519) -> (s? t:f=w535:u16)
        n290 = Subtract(x=w537, y=w536) -> (x-y=w512:u16)
        n291 = Subtract(x=w535, y=w512) -> (x-y=w526:u16)
        n292 = Number To Boolean Array(number=w512) -> (Boolean array=w511:bool[])
        n293 = Or Array Elements(Boolean array=w511) -> (logical OR=w510:bool)
        n294 = Boolean To (0,1)(Boolean="+ phase (APD 2 Gate)") -> (0, 1=w524:i16)
        n295 = Multiply(x=w524, y="Phase count adjustment (APD 2 Gate)") -> (x*y=w522:i16)
        n296 = Boolean To (0,1)(Boolean=w510) -> (0, 1=w517:i16)
        n297 = Add(x=w526, y=w522) -> (x+y=w527:u16)
        n298 = To Unsigned Byte Integer(number=w517) -> (unsigned 8bit integer=w514:u8)
        n299 = feedback #18(i16 0) -> (w529:i16)
        n300 = Subtract(x=w529, y=w522) -> (x-y=w528:i16)
        "APD 2 Gate Relative Phase" <- w528
        n301 = feedback-in #18(w528) -> ()
        n302 = feedback #19(u8 0) -> (w515:u8)
        n303 = Add(x=w514, y=w515) -> (x+y=w513:u8)
        "APD 2 Gate Late Counter" <- w513
        n304 = feedback-in #19(w513) -> ()
        n305 = local read "APD Gate Operating Mode"() -> (w518:u8)
        n306 = case shown="2" w518 {
          tunnel: [TRUE FALSE w544] -> w531
          tunnel: w533 -> [_ _ w542]
          frame 0, Default {
          }
          frame 1 {
          }
          frame 2 {
            n307 = local read "Invert APD Gate"() -> (w541:bool)
            n308 = Not(x=w542) -> (.not. x?=w543:bool)
            n309 = Select(t=w543, s=w541, f=w542) -> (s? t:f=w544:bool)
          }
        }
      }
    }
  }
  n310 = while "532 nm green fluorescent laser interlacing (DO to IA 532 nm AOM ME amp)." {
    shift-right: [w548] -> _
    shift-left: w1 -> [w553]
    shift-right: [w547] -> _
    shift-left: w2 -> [w545]
    stop <- FALSE stop-if-true
    n311 = flat-sequence {
      tunnel: w553 -> [w556]
      tunnel: [w557] -> w551
      tunnel: [w556] -> w549
      tunnel: [w555] -> w546
      tunnel: w545 -> [w555]
      tunnel: [w560] -> w552
      tunnel: w551 -> [w560]
      tunnel: [w559] -> w550
      tunnel: w549 -> [w559]
      tunnel: w546 -> [w558]
      tunnel: [w569] -> w548
      tunnel: w552 -> [w589]
      tunnel: w550 -> [w586]
      tunnel: [w578] -> w547
      frame #0 {
        n312 = call "Loop Timer4"("Count(Ticks)"=w556) -> ("Tick Count(Ticks)"=w557:u16)
      }
      frame #1 {
        # "Then to PRL 440 amp"
        n313 = xnode "FPGA I/O Node"("Connector1/DIO39"=w558) -> ()  [unwired: 1 in, 1 out]
      }
      frame #2 {
        n314 = feedback-in #20(w589) -> ()
        n315 = feedback #20(w589) -> (w588:u16)
        n316 = Subtract(x=w589, y=w588) -> (x-y=w587:u16)
        n317 = Subtract(x=w587, y=w586) -> (x-y=w562:u16)
        n318 = Number To Boolean Array(number=w562) -> (Boolean array=w563:bool[])
        n319 = Or Array Elements(Boolean array=w563) -> (logical OR=w561:bool)
        n320 = Boolean To (0,1)(Boolean="+ phase (GI)") -> (0, 1=w574:i16)
        n321 = Multiply(x=w574, y="Phase count adjustment (GI)") -> (x*y=w571:i16)
        n322 = Boolean To (0,1)(Boolean=w561) -> (0, 1=w568:i16)
        n323 = To Unsigned Byte Integer(number=w568) -> (unsigned 8bit integer=w565:u8)
        n324 = feedback #21(i16 0) -> (w572:i16)
        n325 = feedback #22(u8 0) -> (w566:u8)
        n326 = Add(x=w565, y=w566) -> (x+y=w564:u8)
        "GI Late Counter" <- w564
        n327 = feedback-in #22(w564) -> ()
        n328 = Subtract(x=w572, y=w571) -> (x-y=w570:i16)
        "GI Relative phase" <- w570
        n329 = feedback-in #21(w570) -> ()
        n330 = feedback #23(TRUE) -> (w581:bool)
        n331 = case shown="2" "Operating Mode" {
          tunnel: [TRUE FALSE w595] -> w578
          tunnel: w581 -> [_ _ w592]
          frame 0, Default {
          }
          frame 1 {
          }
          frame 2 {
            n332 = Not(x=w592) -> (.not. x?=w594:bool)
            n333 = Select(t=w594, s="Invert GI", f=w592) -> (s? t:f=w595:bool)
          }
        }
        n334 = Not(x=w581) -> (.not. x?=w577:bool)
        n335 = Select(t="Green interlace ON count", s=w577, f="Green interlace OFF count") -> (s? t:f=w583:u16)
        n336 = Subtract(x=w583, y=w562) -> (x-y=w575:u16)
        n337 = Add(x=w575, y=w571) -> (x+y=w569:u16)
        n338 = feedback-in #23(w577) -> ()
      }
    }
  }
  n339 = while "Green and red fluorescent laser interlacing (Current AO to IA 532 nm AOM ME amp)." {
    shift-right: [w604] -> _
    shift-left: w1 -> [w607]
    shift-right: [w601] -> _
    shift-left: w3 -> [w599]
    shift-right: [w598] -> _
    shift-left: w3 -> [w597]
    stop <- FALSE stop-if-true
    n340 = flat-sequence {
      tunnel: w607 -> [w611]
      tunnel: [w612] -> w606
      tunnel: [w611] -> w605
      tunnel: [w610] -> w600
      tunnel: w599 -> [w610]
      tunnel: w597 -> [w609]
      tunnel: [w609] -> w596
      tunnel: [w616] -> w603
      tunnel: w606 -> [w616]
      tunnel: [w615] -> w602
      tunnel: w605 -> [w615]
      tunnel: w600 -> [w614]
      tunnel: w596 -> [w613]
      tunnel: [w637] -> w604
      tunnel: [w653] -> w601
      tunnel: w603 -> [w664]
      tunnel: w602 -> [w661]
      tunnel: [w621] -> w598
      frame #0 {
        n341 = call "Loop Timer10"("Count(Ticks)"=w611) -> ("Tick Count(Ticks)"=w612:u16)
      }
      frame #1 {
        n342 = xnode "FPGA I/O Node"("Chassis2/Mod4/AO0"=w614, "Chassis2/Mod4/AO1"=w613) -> ()  [unwired: 2 in, 2 out]
      }
      frame #2 {
        # "Design note:\n\nThese two laser controls are in the same loop\nbecause the expansion current AI cannot separately\ntime the outputs fast enough for us.  Apparently\nit is because of communication time between the\nexpansion card and the fpga.\n\nSo the two analog control signals have the same timing\nand profile, but independent amplitudes to independently\ncontrol the intensity and feedback for each laser."
        n343 = feedback #24(TRUE) -> (w617:bool)
        n344 = Not(x=w617) -> (.not. x?=w618:bool)
        n345 = feedback-in #24(w618) -> ()
        n346 = Subtract(x="Green interlace OFF count 2", y="Green int current ON count adj") -> (x-y=w646:u16)
        n347 = feedback-in #25(w664) -> ()
        n348 = feedback #25(w664) -> (w663:u16)
        n349 = Add(x="Green int current ON count adj", y="Green interlace ON count 2") -> (x+y=w647:u16)
        n350 = Subtract(x=w664, y=w663) -> (x-y=w662:u16)
        n351 = Select(t=w647, s=w618, f=w646) -> (s? t:f=w658:u16)
        n352 = Subtract(x=w662, y=w661) -> (x-y=w630:u16)
        n353 = case shown="2" "RI Operating Mode 2" {
          tunnel: [TRUE FALSE w670] -> w619
          tunnel: w617 -> [_ _ w667]
          frame 0, Default {
          }
          frame 1 {
          }
          frame 2 {
            n354 = Not(x=w667) -> (.not. x?=w669:bool)
            n355 = Select(t=w669, s="Invert RI 2", f=w667) -> (s? t:f=w670:bool)
          }
        }
        n356 = Subtract(x=w658, y=w630) -> (x-y=w641:u16)
        n357 = case shown="0, Default" "Operating Mode 2" {
          tunnel: [TRUE FALSE w704] -> w622
          tunnel: w617 -> [_ _ w701]
          frame 0, Default {
          }
          frame 1 {
          }
          frame 2 {
            n358 = Not(x=w701) -> (.not. x?=w703:bool)
            n359 = Select(t=w703, s="Invert GI 2", f=w701) -> (s? t:f=w704:bool)
          }
        }
        n360 = Number To Boolean Array(number=w630) -> (Boolean array=w631:bool[])
        n361 = Boolean To (0,1)(Boolean="+ phase (GI) 2") -> (0, 1=w643:i16)
        n362 = Or Array Elements(Boolean array=w631) -> (logical OR=w629:bool)
        n363 = Boolean To (0,1)(Boolean=w629) -> (0, 1=w636:i16)
        n364 = Multiply(x=w643, y="Phase count adjustment (GI) 2") -> (x*y=w639:i16)
        n365 = To Unsigned Byte Integer(number=w636) -> (unsigned 8bit integer=w632:u8)
        n366 = Add(x=w641, y=w639) -> (x+y=w637:u16)
        n367 = feedback #26(u8 0) -> (w634:u8)
        n368 = Add(x=w632, y=w634) -> (x+y=w633:u8)
        "GI Late Counter 2" <- w633
        n369 = feedback-in #26(w633) -> ()
        n370 = feedback #27(i16 0) -> (w640:i16)
        n371 = Subtract(x=w640, y=w639) -> (x-y=w638:i16)
        "GI Relative phase 2" <- w638
        n372 = feedback-in #27(w638) -> ()
        n373 = And(x=w622, y="Green FB On/Off") -> (x .and. y?=w648:bool)
        n374 = And(x=w619, y="Red FB On/Off") -> (x .and. y?=w628:bool)
        n375 = case shown="True" w648 {
          tunnel: "Current Out" -> [w685 _]
          tunnel: [w685 w694] -> w652
          frame False {
          }
          frame True {
            n376 = local read "Green FB Sum"() -> (w690:i16)
            n377 = Bundle("P3"="P3", "I3"="I3", "D3"="D3") -> (w686:cluster{"P3":i16, "I3":i16, "D3":i16})  [unwired: 1 in]
            n378 = call "Slower PID.vi"("process variable"=w690, "reset?"="Green FB Reset", "setpoint"="Green FB Setpoint", "PID gains (x 2^8)"=w686, "output range"=cluster{"output high":i16, "output low":i16} {"output high"=32767, "output low"=-32768} ("Green FB output range")) -> ("output"=w697:i16)  [unwired: 10 out]
            n379 = To Long Integer(number=w697) -> (32bit integer=w691:i32)
            n380 = Add(x=w691, y=32768) -> (x+y=w693:i32)
            n381 = To Unsigned Word Integer(number=w693) -> (unsigned 16bit integer=w694:u16)
          }
        }
        n382 = case shown="True" w628 {
          tunnel: "RI Current Out" -> [w671 _]
          tunnel: [w671 w680] -> w624
          frame False {
          }
          frame True {
            n383 = local read "Red FB Intensity"() -> (w676:i16)
            n384 = Bundle("P4"="P4", "I4"="I4", "D4"="D4") -> (w672:cluster{"P4":i16, "I4":i16, "D4":i16})  [unwired: 1 in]
            n385 = call "Slower PID.vi"("process variable"=w676, "reset?"="Red FB Reset", "setpoint"="Red FB Setpoint", "PID gains (x 2^8)"=w672, "output range"=cluster{"output high":i16, "output low":i16} {"output high"=32767, "output low"=-32768} ("Green FB output range")) -> ("output"=w683:i16)  [unwired: 10 out]
            n386 = To Long Integer(number=w683) -> (32bit integer=w677:i32)
            n387 = Add(x=w677, y=32768) -> (x+y=w679:i32)
            n388 = To Unsigned Word Integer(number=w679) -> (unsigned 16bit integer=w680:u16)
          }
        }
        n389 = Boolean To (0,1)(Boolean=w622) -> (0, 1=w654:i16)
        n390 = Boolean To (0,1)(Boolean=w619) -> (0, 1=w623:i16)
        n391 = To Unsigned Word Integer(number=w654) -> (unsigned 16bit integer=w651:u16)
        n392 = To Unsigned Word Integer(number=w623) -> (unsigned 16bit integer=w625:u16)
        n393 = Multiply(x=w651, y=w652) -> (x*y=w653:u16)
        n394 = Multiply(x=w625, y=w624) -> (x*y=w621:u16)
      }
    }
  }
  n395 = while "MCL stage control" {
    shift-right: [w717] -> _
    shift-left: w1 -> [w720]
    shift-right: [w710] -> _
    shift-left: w10 -> [w707]
    shift-right: [w709] -> _
    shift-left: w9 -> [w705]
    stop <- FALSE stop-if-true
    n396 = flat-sequence {
      tunnel: w720 -> [w724]
      tunnel: [w725] -> w716
      tunnel: [w724] -> w714
      tunnel: [w723] -> w708
      tunnel: w707 -> [w723]
      tunnel: [w722] -> w706
      tunnel: w705 -> [w722]
      tunnel: w716 -> [w729]
      tunnel: [w729] -> w715
      tunnel: w714 -> [w728]
      tunnel: [w728] -> w713
      tunnel: w708 -> [w727]
      tunnel: w706 -> [w726]
      tunnel: w715 -> [w737]
      tunnel: w713 -> [w736]
      tunnel: [w737] -> w719
      tunnel: [w736] -> w718
      tunnel: [w735] -> w712
      tunnel: [w734] -> w711
      tunnel: [w809] -> w717
      tunnel: w719 -> [w816]
      tunnel: w718 -> [w813]
      tunnel: w712 -> [w811]
      tunnel: w711 -> [w810]
      tunnel: [w811] -> w710
      tunnel: [w810] -> w709
      frame #0 {
        n397 = call "Loop Timer5"("Count(Ticks)"=w724) -> ("Tick Count(Ticks)"=w725:u32)
      }
      frame #1 {
        n398 = xnode "FPGA I/O Node"("Connector0/AO1"=w727, "Connector0/AO2"=w726) -> ()  [unwired: 2 in, 2 out]
      }
      frame #2 {
        n399 = local read "Scanning MCL"() -> (w749:bool)
        n400 = Or(x=w749, y="Start scan (MCL)") -> (x .or. y?=w744:bool)
        n401 = Not(x="Abort scan (MCL)") -> (.not. x?=w742:bool)
        n402 = And(x=w742, y=w744) -> (x .and. y?=w741:bool)
        n403 = case "Raster scan" shown="True" w741 {
          tunnel: [w750 w793] -> w746
          tunnel: "Start scan (MCL)" -> [_ w778]
          tunnel: [w750 w754] -> w730
          frame False {
            w750 = i16 0
            n404 = local write "Scanning MCL"(FALSE ("scanning")) -> ()
          }
          frame True {
            w764 = i16 0
            w763 = u64 0
            # "scan incr."
            # "freq. incr. mult."
            # "count steps"
            # "count number of cycles"
            n405 = feedback #28(w763) -> (w790:u64)
            n406 = Select(t=w763, s=w778, f=w790) -> (s? t:f=w792:u64)
            n407 = Increment(x=w792) -> (x+1=w789:u64)
            n408 = Greater?(x="Cycles per step (MCL)", y=w789) -> (0:w773:bool)
            n409 = Select(t=w789, s=w773, f=w763) -> (s? t:f=w788:u64)
            n410 = feedback-in #28(w788) -> ()
            n411 = feedback #29(w763) -> (w787:u64)
            n412 = Select(t=w763, s=w778, f=w787) -> (s? t:f=w782:u64)
            n413 = Increment(x=w782) -> (x+1=w786:u64)
            n414 = Add(x="Scan steps (MCL)", y="Scan steps (MCL)") -> (x+y=w785:u64)
            n415 = Select(t=w782, s=w773, f=w786) -> (s? t:f=w768:u64)
            n416 = Greater?(x=w785, y=w768) -> (0:w767:bool)
            n417 = Select(t=w768, s=w767, f=w763) -> (s? t:f=w783:u64)
            n418 = feedback-in #29(w783) -> ()
            n419 = Equal?(x="Scan steps (MCL)", y=w768) -> (x = y?=w772:bool)
            n420 = Greater?(x="Scan steps (MCL)", y=w782) -> (0:w781:bool)
            n421 = feedback #30(w764) -> (w784:i16)
            n422 = Select(t=w764, s=w778, f=w784) -> (s? t:f=w770:i16)
            n423 = Increment(x=w770) -> (x+1=w780:i16)
            n424 = Decrement(x=w770) -> (x-1=w779:i16)
            n425 = Select(t=w780, s=w781, f=w779) -> (s? t:f=w771:i16)
            n426 = Select(t=w770, s=w772, f=w771) -> (s? t:f=w769:i16)
            n427 = Select(t=w770, s=w773, f=w769) -> (s? t:f=w765:i16)
            n428 = Select(t=w765, s=w767, f=w764) -> (s? t:f=w766:i16)
            n429 = feedback-in #30(w766) -> ()
            n430 = feedback #31(w763) -> (w777:u64)
            n431 = Select(t=w763, s=w778, f=w777) -> (s? t:f=w752:u64)
            n432 = Increment(x=w752) -> (x+1=w774:u64)
            n433 = Select(t=w752, s=w767, f=w774) -> (s? t:f=w753:u64)
            n434 = Greater?(x="Number of scans (MCL)", y=w753) -> (0:w760:bool)
            n435 = Multiply(x="Scan freq.  increment (MCL)", y=w770) -> (x*y=w793:i16)
            n436 = Select(t=TRUE, s="Cont. Scan (MCL)", f=w760) -> (s? t:f=w759:bool)
            "Scanning MCL" <- w759
            n437 = Select(t=w753, s=w759, f=w763) -> (s? t:f=w775:u64)
            n438 = feedback-in #31(w775) -> ()
            n439 = Increment(x=w753) -> (x+1=→"Scan I (MCL)":u64)
            n440 = To Word Integer(number=w752) -> (16bit integer=w755:i16)
            n441 = Multiply(x=w755, y="Scan freq.  increment (MCL)") -> (x*y=w754:i16)
          }
        }
        n442 = Select(t=w730, s="1D or 2D Scan?", f=i16 0) -> (s? t:f=w731:i16)
        n443 = Select(t=w731, s="MCL Scan Axis", f=w746) -> (s? t:f=w745:i16)
        n444 = Select(t=w746, s="MCL Scan Axis", f=w731) -> (s? t:f=w747:i16)
        n445 = Add(x=w745, y="AO2") -> (x+y=w734:i16)
        n446 = Add(x="AO1", y=w747) -> (x+y=w735:i16)
      }
      frame #3 {
        n447 = feedback-in #32(w816) -> ()
        n448 = feedback #32(w816) -> (w815:u32)
        n449 = Boolean To (0,1)(Boolean="+ phase (MCL)") -> (0, 1=w807:i16)
        n450 = Subtract(x=w816, y=w815) -> (x-y=w814:u32)
        n451 = Multiply(x=w807, y="Phase count adjustment (MCL)") -> (x*y=w803:i16)
        n452 = Subtract(x=w814, y=w813) -> (x-y=w795:u32)
        n453 = Subtract(x="MCL count", y=w795) -> (x-y=w805:u32)
        n454 = feedback #33(i16 0) -> (w804:i16)
        n455 = Subtract(x=w804, y=w803) -> (x-y=w802:i16)
        "MCL Relative Phase" <- w802
        n456 = feedback-in #33(w802) -> ()
        n457 = Number To Boolean Array(number=w795) -> (Boolean array=w796:bool[])
        n458 = Or Array Elements(Boolean array=w796) -> (logical OR=w794:bool)
        n459 = Boolean To (0,1)(Boolean=w794) -> (0, 1=w801:i16)
        n460 = Add(x=w805, y=w803) -> (x+y=w809:u32)
        n461 = To Unsigned Byte Integer(number=w801) -> (unsigned 8bit integer=w798:u8)
        n462 = feedback #34(u8 0) -> (w799:u8)
        n463 = Add(x=w798, y=w799) -> (x+y=w797:u8)
        "MCL Late Counter" <- w797
        n464 = feedback-in #34(w797) -> ()
      }
    }
  }
  n465 = while "Excitation laser intensity feedback measurement (all lasers)" {
    shift-right: [w818] -> _
    shift-left: w1 -> [w823]
    stop <- FALSE stop-if-true
    n466 = flat-sequence {
      tunnel: w823 -> [w825]
      tunnel: [w826] -> w821
      tunnel: [w825] -> w819
      tunnel: [w832] -> w822
      tunnel: w821 -> [w832]
      tunnel: [w831] -> w820
      tunnel: w819 -> [w831]
      tunnel: [w844] -> w818
      tunnel: w822 -> [w855]
      tunnel: w820 -> [w852]
      frame #0 {
        n467 = call "Loop Timer9"("Count(Ticks)"=w825) -> ("Tick Count(Ticks)"=w826:u16)
      }
      frame #1 {
        # "Design note:\n\nAll lasers need to be measured at the same \ntime because the AI expansion module\ncannot independently time the measurements\nwithin our requirements: their is dead time.\n\nThis probably wouldn't be an issue with the built\nin AI on the fpga board itself."
        n468 = xnode "FPGA I/O Node"("Connector1/DIO35"=TRUE) -> ("Chassis2/Mod1/AI2"=→"Blue Intensity":i16, "Chassis2/Mod1/AI1"=→"Red FB Intensity":i16, "Chassis2/Mod1/AI0"=→"Green FB Sum":i16)  [unwired: 4 in, 4 out]
      }
      frame #2 {
        n469 = feedback-in #35(w855) -> ()
        n470 = feedback #35(w855) -> (w854:u16)
        n471 = Subtract(x=w855, y=w854) -> (x-y=w853:u16)
        n472 = xnode "FPGA I/O Node"("Connector1/DIO35"=FALSE) -> ()  [unwired: 1 in, 1 out]
        n473 = Subtract(x=w853, y=w852) -> (x-y=w834:u16)
        n474 = Subtract(x="Green FB Count", y=w834) -> (x-y=w848:u16)
        n475 = Number To Boolean Array(number=w834) -> (Boolean array=w835:bool[])
        n476 = Or Array Elements(Boolean array=w835) -> (logical OR=w833:bool)
        n477 = Boolean To (0,1)(Boolean="+ phase (Green FB)") -> (0, 1=w846:i16)
        n478 = Boolean To (0,1)(Boolean=w833) -> (0, 1=w840:i16)
        n479 = Multiply(x=w846, y="Phase count adjustment (Green FB)") -> (x*y=w841:i16)
        n480 = Add(x=w848, y=w841) -> (x+y=w844:u16)
        n481 = To Unsigned Byte Integer(number=w840) -> (unsigned 8bit integer=w837:u8)
        n482 = feedback #36(i16 0) -> (w843:i16)
        n483 = Subtract(x=w843, y=w841) -> (x-y=w842:i16)
        "Green FB Relative Phase" <- w842
        n484 = feedback-in #36(w842) -> ()
        n485 = feedback #37(u8 0) -> (w838:u8)
        n486 = Add(x=w837, y=w838) -> (x+y=w836:u8)
        "Green Late Counter" <- w836
        n487 = feedback-in #37(w836) -> ()
      }
    }
  }
  n488 = while "APD 1 Gating" {
    shift-right: [w859] -> _
    shift-left: w1 -> [w864]
    shift-right: [w858] -> _
    shift-left: w5 -> [w856]
    stop <- FALSE stop-if-true
    n489 = flat-sequence {
      tunnel: w864 -> [w867]
      tunnel: [w868] -> w862
      tunnel: [w867] -> w860
      tunnel: [w866] -> w857
      tunnel: w856 -> [w866]
      tunnel: [w871] -> w863
      tunnel: w862 -> [w871]
      tunnel: [w870] -> w861
      tunnel: w860 -> [w870]
      tunnel: w857 -> [w869]
      tunnel: [w885] -> w859
      tunnel: w863 -> [w900]
      tunnel: w861 -> [w897]
      tunnel: [w889] -> w858
      frame #0 {
        n490 = call "Loop Timer7"("Count(Ticks)"=w867) -> ("Tick Count(Ticks)"=w868:u16)
      }
      frame #1 {
        # "Signal is then sent through \na transistor before APD"
        n491 = xnode "FPGA I/O Node"("Connector0/DIO4"=w869) -> ()  [unwired: 1 in, 1 out]
      }
      frame #2 {
        n492 = feedback #38(TRUE) -> (w892:bool)
        n493 = feedback-in #39(w900) -> ()
        n494 = feedback #39(w900) -> (w899:u16)
        n495 = Not(x=w892) -> (.not. x?=w888:bool)
        n496 = feedback-in #38(w888) -> ()
        n497 = Subtract(x=w900, y=w899) -> (x-y=w898:u16)
        n498 = Select(t="APD Gate ON Count", s=w888, f="APD Gate OFF Count") -> (s? t:f=w894:u16)
        n499 = Subtract(x=w898, y=w897) -> (x-y=w873:u16)
        n500 = Subtract(x=w894, y=w873) -> (x-y=w884:u16)
        n501 = Number To Boolean Array(number=w873) -> (Boolean array=w874:bool[])
        n502 = Or Array Elements(Boolean array=w874) -> (logical OR=w872:bool)
        n503 = Boolean To (0,1)(Boolean="+ phase (APD 1 Gate)") -> (0, 1=w882:i16)
        n504 = Boolean To (0,1)(Boolean=w872) -> (0, 1=w879:i16)
        n505 = Multiply(x=w882, y="Phase count adjustment (APD 1 Gate)") -> (x*y=w880:i16)
        n506 = To Unsigned Byte Integer(number=w879) -> (unsigned 8bit integer=w876:u8)
        n507 = Add(x=w884, y=w880) -> (x+y=w885:u16)
        n508 = feedback #40(i16 0) -> (w887:i16)
        n509 = Subtract(x=w887, y=w880) -> (x-y=w886:i16)
        "APD 1 Gate Relative Phase" <- w886
        n510 = feedback-in #40(w886) -> ()
        n511 = feedback #41(u8 0) -> (w877:u8)
        n512 = Add(x=w876, y=w877) -> (x+y=w875:u8)
        "APD 1 Gate Late Counter" <- w875
        n513 = feedback-in #41(w875) -> ()
        n514 = case shown="2" "APD Gate Operating Mode" {
          tunnel: [TRUE FALSE w906] -> w889
          tunnel: w892 -> [_ _ w903]
          frame 0, Default {
          }
          frame 1 {
          }
          frame 2 {
            n515 = Not(x=w903) -> (.not. x?=w905:bool)
            n516 = Select(t=w905, s="Invert APD Gate", f=w903) -> (s? t:f=w906:bool)
          }
        }
      }
    }
  }
  n517 = while "Control APD data integration - stream to host" {
    shift-right: [w910] -> _
    shift-left: w6 -> [w915]
    stop <- FALSE stop-if-true
    n518 = flat-sequence {
      tunnel: w915 -> [w917]
      tunnel: [w918] -> w913
      tunnel: [w917] -> w911
      tunnel: [w928] -> w914
      tunnel: w913 -> [w928]
      tunnel: [w927] -> w912
      tunnel: w911 -> [w927]
      tunnel: [w926] -> w909
      tunnel: [w925] -> w908
      tunnel: [w919] -> w907
      tunnel: [w970] -> w910
      tunnel: w914 -> [w980]
      tunnel: w912 -> [w977]
      tunnel: w909 -> [w963]
      tunnel: w908 -> [w962]
      tunnel: w907 -> [w950]
      frame #0 {
        n519 = call "Loop Timer6"("Count(Ticks)"=w917) -> ("Tick Count(Ticks)"=w918:u32)
      }
      frame #1 {
        n520 = flat-sequence {
          tunnel: [w930] -> w924
          tunnel: w924 -> [w933]
          tunnel: [w937] -> w923
          tunnel: [w936] -> w922
          tunnel: [w933] -> w921
          tunnel: [w932] -> w920
          tunnel: [w944] -> w925
          tunnel: [w945] -> w926
          tunnel: w923 -> [w945]
          tunnel: w922 -> [w944]
          tunnel: w921 -> [w943]
          tunnel: w920 -> [w942]
          tunnel: [w942] -> w919
          frame #0 {
            # "use separate variable so each APD won't\nhave to wait to read"
            n521 = feedback #42(FALSE) -> (w929:bool)
            "APD1 out state" <- w929
            "APD2 out state" <- w929
            "APD3 out state" <- w929
            n522 = Not(x=w929) -> (.not. x?=w930:bool)
            n523 = feedback-in #42(w930) -> ()
          }
          frame #1 {
            n524 = local read "APD 3 Counts 1"() -> (w935:u32)
            n525 = local read "APD 3 Counts 0"() -> (w934:u32)
            n526 = local read "APD 1 Counts 1"() -> (w941:u32)
            n527 = local read "APD 1 Counts 0"() -> (w940:u32)
            n528 = local read "APD 2 Counts 1"() -> (w939:u32)
            n529 = local read "APD 2 Counts 0"() -> (w938:u32)
            n530 = Select(t=w935, s=w933, f=w934) -> (s? t:f=w932:u32)
            n531 = Select(t=w941, s=w933, f=w940) -> (s? t:f=w937:u32)
            n532 = Select(t=w939, s=w933, f=w938) -> (s? t:f=w936:u32)
          }
          frame #2 {
            n533 = case shown="False" w943 {
              frame False {
                w946 = u32 0 ("APD 1 Counts 0")
                n534 = local write "APD 1 Counts 0"(w946) -> ()
                n535 = local write "APD 2 Counts 0"(w946) -> ()
                n536 = local write "APD 3 Counts 0"(w946) -> ()
              }
              frame True {
                w947 = u32 0 ("APD 1 Counts 1")
                n537 = local write "APD 1 Counts 1"(w947) -> ()
                n538 = local write "APD 2 Counts 1"(w947) -> ()
                n539 = local write "APD 3 Counts 1"(w947) -> ()
              }
            }
          }
        }
      }
      frame #2 {
        n540 = feedback-in #43(w980) -> ()
        n541 = feedback #43(w980) -> (w979:u32)
        n542 = Subtract(x=w980, y=w979) -> (x-y=w978:u32)
        n543 = Subtract(x=w978, y=w977) -> (x-y=w955:u32)
        n544 = case shown="True" "APD to FIFO" {
          tunnel: w963 -> [_ w985]
          tunnel: w962 -> [_ w983]
          tunnel: w950 -> [_ w981]
          frame False {
          }
          frame True {
            n545 = flat-sequence {
              tunnel: 0 ("Timeout") -> [w987]
              tunnel: w985 -> [w988]
              tunnel: [w987] -> w984
              tunnel: w984 -> [w989]
              tunnel: w983 -> [w990]
              tunnel: [w989] -> w982
              tunnel: w982 -> [w992]
              tunnel: w981 -> [w991]
              frame #0 {
                n546 = xnode ("FIFO Write")("Element"=w988, "Timeout"=w987) -> ()  [unwired: 1 in, 2 out]
              }
              frame #1 {
                n547 = xnode ("FIFO Write")("Element"=w990, "Timeout"=w989) -> ()  [unwired: 1 in, 2 out]
              }
              frame #2 {
                n548 = xnode ("FIFO Write")("Element"=w991, "Timeout"=w992) -> ()  [unwired: 1 in, 2 out]
              }
            }
          }
        }
        n549 = Subtract(x="APD Acq Rate Count", y=w955) -> (x-y=w971:u32)
        n550 = Number To Boolean Array(number=w955) -> (Boolean array=w956:bool[])
        n551 = Or Array Elements(Boolean array=w956) -> (logical OR=w954:bool)
        n552 = Boolean To (0,1)(Boolean=w954) -> (0, 1=w961:i16)
        n553 = To Unsigned Byte Integer(number=w961) -> (unsigned 8bit integer=w958:u8)
        n554 = feedback #44(u8 0) -> (w959:u8)
        n555 = Add(x=w958, y=w959) -> (x+y=w957:u8)
        "APD Acq Late Counter" <- w957
        n556 = feedback-in #44(w957) -> ()
        n557 = Boolean To (0,1)(Boolean="+ phase (APD Acq)") -> (0, 1=w967:i16)
        n558 = Multiply(x=w967, y="Phase Count Adjustment (APD Acq)") -> (x*y=w964:i16)
        n559 = Add(x=w971, y=w964) -> (x+y=w970:u32)
        n560 = feedback #45(i16 0) -> (w969:i16)
        n561 = Subtract(x=w969, y=w964) -> (x-y=w966:i16)
        "APD Acq Relative Phase" <- w966
        n562 = feedback-in #45(w966) -> ()
        n563 = To Word Integer(number=w963) -> (16bit integer=w972:i16)
        n564 = To Word Integer(number=w950) -> (16bit integer=w951:i16)
        n565 = To Word Integer(number=w962) -> (16bit integer=w973:i16)
        n566 = Multiply(x="APD AO scale factor", y=w973) -> (x*y=w952:i16)
        n567 = Multiply(x="APD AO scale factor", y=w951) -> (x*y=w948:i16)
        n568 = Multiply(x="APD AO scale factor", y=w972) -> (x*y=w953:i16)
        n569 = xnode "FPGA I/O Node"("Connector0/AO5"=w953, "Connector0/AO7"=w952, "Connector0/AO6"=w948) -> ()  [unwired: 3 in, 3 out]
      }
    }
  }
  n570 = while "DAQ AI set 1" {
    shift-right: [w993] -> _
    shift-left: w1 -> [w998]
    stop <- FALSE stop-if-true
    n571 = flat-sequence {
      tunnel: w998 -> [w1008]
      tunnel: [w1009] -> w996
      tunnel: [w1008] -> w995
      tunnel: [w1019] -> w1006
      tunnel: [w1018] -> w1005
      tunnel: [w1017] -> w1004
      tunnel: [w1016] -> w1003
      tunnel: [w1015] -> w1002
      tunnel: [w1014] -> w1001
      tunnel: [w1013] -> w1000
      tunnel: [w1012] -> w999
      tunnel: [w1011] -> w997
      tunnel: w996 -> [w1011]
      tunnel: w995 -> [w1010]
      tunnel: [w1010] -> w994
      tunnel: [w1048] -> w993
      tunnel: w1006 -> [w1075]
      tunnel: w1005 -> [w1040]
      tunnel: w1004 -> [w1041]
      tunnel: w1003 -> [w1074]
      tunnel: w1002 -> [w1064]
      tunnel: w1001 -> [w1063]
      tunnel: w1000 -> [w1062]
      tunnel: w999 -> [w1061]
      tunnel: w997 -> [w1058]
      tunnel: w994 -> [w1055]
      frame #0 {
        n572 = call "Loop Timer3"("Count(Ticks)"=w1008) -> ("Tick Count(Ticks)"=w1009:u16)
      }
      frame #1 {
        n573 = xnode "FPGA I/O Node"("Connector1/DIO31"=TRUE ("Connector1/DIO33")) -> ("Connector0/AI0"=w1019:i16, "Connector0/AI1"=w1018:i16, "Connector0/AI2"=w1017:i16, "Connector0/AI3"=w1016:i16, "Connector0/AI4"=w1015:i16, "Connector0/AI5"=w1014:i16, "Connector0/AI6"=w1013:i16, "Connector0/AI7"=w1012:i16)  [unwired: 9 in, 9 out]
      }
      frame #2 {
        w1044 = FALSE ("AI to FIFO")
        # "Adjust phase after data acquired if button pressed"
        n574 = feedback #46(i16 1) -> (w1067:i16)
        n575 = Increment(x=w1067) -> (x+1=w1073:i16)
        n576 = Scale By Power Of 2(n="AI1 X Scale", x=w1040) -> (x*2^n=w1038:i16)
        n577 = Greater?(x=w1073, y="N of AI1 Int Acq Sets") -> (0:w1070:bool)
        n578 = Select(t=i16 1, s=w1070, f=w1073) -> (s? t:f=w1072:i16)
        n579 = feedback-in #46(w1072) -> ()
        n580 = Divide(x=w1038, y=w1041) -> (x/y=w1037:fxp<+/-,16,1>)
        n581 = feedback #47(w1044) -> (w1042:bool)
        n582 = feedback #48(w1044) -> (w1060:bool)
        n583 = case shown="2" w1067 {
          tunnel: w1041 -> [w1098 w1105 _]
          tunnel: ["Set 1" "Set 2" "Set 3"] -> w1065
          tunnel: ["AI to FIFO" w1107 w1112] -> w1059
          tunnel: w1060 -> [_ w1107 w1112]
          tunnel: ["Trap Pos to FIFO" w1106 w1111] -> w1043
          tunnel: w1042 -> [_ w1106 w1111]
          tunnel: w1037 -> [w1097 w1104 _]
          tunnel: [w1096 w1102 FALSE] -> w1024
          tunnel: [w1095 w1103 u64 0 ("BD1 Frequency Out 2")] -> w1023
          frame 1, Default {
            n584 = local read "BD1 Frequency Out 1"() -> (w1095:u64)
            n585 = Compound Arithmetic op=AND("Trap Pos to FIFO", "Set 1", "AI to FIFO") -> (w1096:bool)
            "AI2 Y Sum Set 1" <- w1098
            "AI1 X Set 1" <- w1097
          }
          frame 2 {
            n586 = local read "BD1 Frequency Out 2"() -> (w1103:u64)
            n587 = Compound Arithmetic op=AND(w1106, "Set 2", w1107) -> (w1102:bool)
            "AI2 Y Sum Set 2" <- w1105
            "AI1 X Set 2" <- w1104
          }
          frame 3 {
          }
        }
        n588 = And(x=w1065, y=w1059) -> (x .and. y?=w1066:bool)
        n589 = case shown="True" w1066 {
          tunnel: w1075 -> [_ w1126]
          tunnel: w1040 -> [_ w1125]
          tunnel: w1041 -> [_ w1124]
          tunnel: w1074 -> [_ w1123]
          tunnel: w1064 -> [_ w1122]
          tunnel: w1063 -> [_ w1121]
          tunnel: w1062 -> [_ w1120]
          tunnel: w1061 -> [_ w1119]
          tunnel: 0 ("DMA buffer timeout") -> [_ w1128]
          frame False {
          }
          frame True {
            n590 = Build Array(w1126, w1125, w1124, w1123, w1122, w1121, w1120, w1119) -> (w1127:i16[])
            n591 = for {
              tunnel: w1127 -> [w1130] mode=indexing
              tunnel: w1128 -> [w1131]
              tunnel: [w1129] -> w1117 mode=indexing
              n592 = xnode ("FIFO Write")("Element"=w1130, "Timeout"=w1131) -> ("Timed Out?"=w1129:bool)  [unwired: 1 in, 1 out]
            }
            n593 = Or Array Elements(Boolean array=w1117) -> (logical OR=w1114:bool)
            n594 = Boolean To (0,1)(Boolean=w1114) -> (0, 1=w1116:i16)
            n595 = feedback #49(u16 0) -> (w1115:u16)
            n596 = Add(x=w1116, y=w1115) -> (x+y=w1113:u16)
            "Trap AI FIFO Timeout" <- w1113
            n597 = feedback-in #49(w1113) -> ()
          }
        }
        n598 = feedback-in #47(w1043) -> ()
        n599 = feedback-in #48(w1059) -> ()
        n600 = case shown="True" w1024 {
          tunnel: w1023 -> [_ w1081]
          tunnel: [u8 0 w1078] -> w1022
          frame False {
          }
          frame True {
            n601 = Split Number(x=w1081) -> (hi(x)=w1082:u32, lo(x)=w1083:u32)
            n602 = Split Number(x=w1082) -> (lo(x)=w1084:u16)  [unwired: 1 out]
            n603 = Split Number(x=w1083) -> (hi(x)=w1085:u16, lo(x)=w1086:u16)
            n604 = Build Array "BD 1 nu Stack"(w1084, w1085, w1086) -> (w1080:u16[])
            n605 = for {
              tunnel: w1080 -> [w1093] mode=indexing
              shift-right: [w1089] -> w1078
              shift-left: u8 0 -> [w1090]
              n606 = xnode ("FIFO Method Node")("Element"=w1093, "Timeout"="Trap FIFO Set Timeout") -> ("Timed Out?"=w1092:bool)  [unwired: 1 in, 1 out]
              n607 = Boolean To (0,1)(Boolean=w1092) -> (0, 1=w1091:i16)
              n608 = To Unsigned Byte Integer(number=w1091) -> (unsigned 8bit integer=w1088:u8)
              n609 = Add(x=w1088, y=w1090) -> (x+y=w1089:u8)
            }
          }
        }
        n610 = To Unsigned Word Integer(number=w1022) -> (unsigned 16bit integer=w1021:u16)
        n611 = feedback #50(u16 0) -> (w1035:u16)
        n612 = Add(x=w1021, y=w1035) -> (x+y=w1034:u16)
        "Trap Pos FIFO Timeout" <- w1034
        n613 = feedback-in #50(w1034) -> ()
        n614 = feedback-in #51(w1058) -> ()
        n615 = feedback #51(w1058) -> (w1057:u16)
        n616 = Subtract(x=w1058, y=w1057) -> (x-y=w1056:u16)
        n617 = xnode "FPGA I/O Node"("Connector1/DIO31"=FALSE ("Connector1/DIO34")) -> ()  [unwired: 1 in, 1 out]
        n618 = Subtract(x=w1056, y=w1055) -> (x-y=w1026:u16)
        n619 = Boolean To (0,1)(Boolean="+ phase") -> (0, 1=w1051:i16)
        n620 = Multiply(x=w1051, y="Phase count adjustment") -> (x*y=w1045:i16)
        n621 = Subtract(x="ai count", y=w1026) -> (x-y=w1049:u16)
        n622 = Number To Boolean Array(number=w1026) -> (Boolean array=w1027:bool[])
        n623 = feedback #52(i16 0) -> (w1047:i16)
        n624 = Add(x=w1049, y=w1045) -> (x+y=w1048:u16)
        n625 = Subtract(x=w1047, y=w1045) -> (x-y=w1046:i16)
        "Relative phase" <- w1046
        n626 = feedback-in #52(w1046) -> ()
        n627 = Or Array Elements(Boolean array=w1027) -> (logical OR=w1025:bool)
        n628 = Boolean To (0,1)(Boolean=w1025) -> (0, 1=w1032:i16)
        n629 = To Unsigned Byte Integer(number=w1032) -> (unsigned 8bit integer=w1029:u8)
        n630 = feedback #53(u8 0) -> (w1030:u8)
        n631 = Add(x=w1029, y=w1030) -> (x+y=w1028:u8)
        "AI Late Counter" <- w1028
        n632 = feedback-in #53(w1028) -> ()
      }
    }
  }
  n633 = node-c288(w7) -> ()
  n634 = while "APD 3 Counter" {
    tunnel: w1 -> [_]
    stop <- FALSE stop-if-true
    n635 = flat-sequence {
      frame #0 {
        n636 = xnode "FPGA I/O Method Node"("FPGA I/O In"=refnum<k21> "Connector0/DIO2" ("APD 2 DO"), "Timeout"=-1) -> ()  [unwired: 2 out]
      }
      frame #1 {
        n637 = local read "APD3 out state"() -> (w1135:bool)
        n638 = case shown="False" w1135 {
          frame False {
            n639 = local read "APD 3 Counts 0"() -> (w1137:u32)
            n640 = Increment(x=w1137) -> (x+1=→"APD 3 Counts 0":u32)
          }
          frame True {
            n641 = local read "APD 3 Counts 1"() -> (w1139:u32)
            n642 = Increment(x=w1139) -> (x+1=→"APD 3 Counts 1":u32)
          }
        }
      }
    }
  }
  n643 = while "APD 3 Gating" {
    shift-right: [w1143] -> _
    shift-left: w1 -> [w1148]
    shift-right: [w1142] -> _
    shift-left: w5 -> [w1140]
    stop <- FALSE stop-if-true
    n644 = flat-sequence {
      tunnel: w1148 -> [w1151]
      tunnel: [w1152] -> w1146
      tunnel: [w1151] -> w1144
      tunnel: [w1150] -> w1141
      tunnel: w1140 -> [w1150]
      tunnel: [w1155] -> w1147
      tunnel: w1146 -> [w1155]
      tunnel: [w1154] -> w1145
      tunnel: w1144 -> [w1154]
      tunnel: w1141 -> [w1153]
      tunnel: [w1172] -> w1143
      tunnel: w1147 -> [w1184]
      tunnel: w1145 -> [w1181]
      tunnel: [w1176] -> w1142
      frame #0 {
        n645 = call "Loop Timer15"("Count(Ticks)"=w1151) -> ("Tick Count(Ticks)"=w1152:u16)
      }
      frame #1 {
        # "Signal is then sent through \na transistor before APD"
        n646 = xnode "FPGA I/O Node"("Connector0/DIO9"=w1153) -> ()  [unwired: 1 in, 1 out]
      }
      frame #2 {
        n647 = local read "APD Gate OFF Count"() -> (w1157:u16)
        n648 = local read "APD Gate ON Count"() -> (w1158:u16)
        n649 = feedback #54(TRUE) -> (w1178:bool)
        n650 = feedback-in #55(w1184) -> ()
        n651 = feedback #55(w1184) -> (w1183:u16)
        n652 = Not(x=w1178) -> (.not. x?=w1175:bool)
        n653 = feedback-in #54(w1175) -> ()
        n654 = Subtract(x=w1184, y=w1183) -> (x-y=w1182:u16)
        n655 = Select(t=w1158, s=w1175, f=w1157) -> (s? t:f=w1180:u16)
        n656 = Subtract(x=w1182, y=w1181) -> (x-y=w1160:u16)
        n657 = Subtract(x=w1180, y=w1160) -> (x-y=w1171:u16)
        n658 = Number To Boolean Array(number=w1160) -> (Boolean array=w1161:bool[])
        n659 = Or Array Elements(Boolean array=w1161) -> (logical OR=w1159:bool)
        n660 = Boolean To (0,1)(Boolean=w1159) -> (0, 1=w1166:i16)
        n661 = Boolean To (0,1)(Boolean="+ phase (APD 3 Gate)") -> (0, 1=w1169:i16)
        n662 = To Unsigned Byte Integer(number=w1166) -> (unsigned 8bit integer=w1163:u8)
        n663 = Multiply(x=w1169, y="Phase count adjustment (APD 3 Gate)") -> (x*y=w1167:i16)
        n664 = feedback #56(u8 0) -> (w1164:u8)
        n665 = Add(x=w1163, y=w1164) -> (x+y=w1162:u8)
        "APD 3 Gate Late Counter" <- w1162
        n666 = feedback-in #56(w1162) -> ()
        n667 = Add(x=w1171, y=w1167) -> (x+y=w1172:u16)
        n668 = feedback #57(i16 0) -> (w1174:i16)
        n669 = Subtract(x=w1174, y=w1167) -> (x-y=w1173:i16)
        "APD 3 Gate Relative Phase" <- w1173
        n670 = feedback-in #57(w1173) -> ()
        n671 = local read "APD Gate Operating Mode"() -> (w1156:u8)
        n672 = case shown="2" w1156 {
          tunnel: [TRUE FALSE w1190] -> w1176
          tunnel: w1178 -> [_ _ w1188]
          frame 0, Default {
          }
          frame 1 {
          }
          frame 2 {
            n673 = local read "Invert APD Gate"() -> (w1187:bool)
            n674 = Not(x=w1188) -> (.not. x?=w1189:bool)
            n675 = Select(t=w1189, s=w1187, f=w1188) -> (s? t:f=w1190:bool)
          }
        }
      }
    }
  }
  n676 = while "633 nm red  fluorescent laser interlacing (DO to IA 633 nm AOM ME amp)." {
    shift-right: [w1194] -> _
    shift-left: w1 -> [w1199]
    shift-right: [w1193] -> _
    shift-left: w2 -> [w1191]
    stop <- FALSE stop-if-true
    n677 = flat-sequence {
      tunnel: w1199 -> [w1202]
      tunnel: [w1203] -> w1197
      tunnel: [w1202] -> w1195
      tunnel: [w1201] -> w1192
      tunnel: w1191 -> [w1201]
      tunnel: [w1206] -> w1198
      tunnel: w1197 -> [w1206]
      tunnel: [w1205] -> w1196
      tunnel: w1195 -> [w1205]
      tunnel: w1192 -> [w1204]
      tunnel: [w1215] -> w1194
      tunnel: w1198 -> [w1235]
      tunnel: w1196 -> [w1232]
      tunnel: [w1224] -> w1193
      frame #0 {
        n678 = call "Loop Timer11"("Count(Ticks)"=w1202) -> ("Tick Count(Ticks)"=w1203:u16)
      }
      frame #1 {
        # "Then to PRL 440 amp"
        n679 = xnode "FPGA I/O Node"("Connector1/DIO32"=w1204) -> ()  [unwired: 1 in, 1 out]
      }
      frame #2 {
        n680 = feedback-in #58(w1235) -> ()
        n681 = feedback #58(w1235) -> (w1234:u16)
        n682 = Subtract(x=w1235, y=w1234) -> (x-y=w1233:u16)
        n683 = Subtract(x=w1233, y=w1232) -> (x-y=w1208:u16)
        n684 = Number To Boolean Array(number=w1208) -> (Boolean array=w1209:bool[])
        n685 = Or Array Elements(Boolean array=w1209) -> (logical OR=w1207:bool)
        n686 = Boolean To (0,1)(Boolean="+ phase (RI)") -> (0, 1=w1220:i16)
        n687 = Multiply(x=w1220, y="Phase count adjustment (RI)") -> (x*y=w1217:i16)
        n688 = Boolean To (0,1)(Boolean=w1207) -> (0, 1=w1214:i16)
        n689 = To Unsigned Byte Integer(number=w1214) -> (unsigned 8bit integer=w1211:u8)
        n690 = feedback #59(i16 0) -> (w1218:i16)
        n691 = feedback #60(u8 0) -> (w1212:u8)
        n692 = Add(x=w1211, y=w1212) -> (x+y=w1210:u8)
        "RI Late Counter" <- w1210
        n693 = feedback-in #60(w1210) -> ()
        n694 = Subtract(x=w1218, y=w1217) -> (x-y=w1216:i16)
        "RI Relative phase" <- w1216
        n695 = feedback-in #59(w1216) -> ()
        n696 = feedback #61(TRUE) -> (w1227:bool)
        n697 = case shown="2" "Red Laser Operating Mode" {
          tunnel: [TRUE FALSE w1241] -> w1224
          tunnel: w1227 -> [_ _ w1238]
          frame 0, Default {
          }
          frame 1 {
          }
          frame 2 {
            n698 = Not(x=w1238) -> (.not. x?=w1240:bool)
            n699 = Select(t=w1240, s="Invert RI", f=w1238) -> (s? t:f=w1241:bool)
          }
        }
        n700 = Not(x=w1227) -> (.not. x?=w1223:bool)
        n701 = Select(t="Red interlace ON count", s=w1223, f="Red interlace OFF count") -> (s? t:f=w1229:u16)
        n702 = Subtract(x=w1229, y=w1208) -> (x-y=w1221:u16)
        n703 = Add(x=w1221, y=w1217) -> (x+y=w1215:u16)
        n704 = feedback-in #61(w1223) -> ()
      }
    }
  }
  n705 = while "473 nm blue  fluorescent laser interlacing (DO to blue laser digital control input)." {
    shift-right: [w1245] -> _
    shift-left: w1 -> [w1250]
    shift-right: [w1244] -> _
    shift-left: w2 -> [w1242]
    stop <- FALSE stop-if-true
    n706 = flat-sequence {
      tunnel: w1250 -> [w1253]
      tunnel: [w1254] -> w1248
      tunnel: [w1253] -> w1246
      tunnel: [w1252] -> w1243
      tunnel: w1242 -> [w1252]
      tunnel: [w1257] -> w1249
      tunnel: w1248 -> [w1257]
      tunnel: [w1256] -> w1247
      tunnel: w1246 -> [w1256]
      tunnel: w1243 -> [w1255]
      tunnel: [w1266] -> w1245
      tunnel: w1249 -> [w1286]
      tunnel: w1247 -> [w1283]
      tunnel: [w1275] -> w1244
      frame #0 {
        n707 = call "Loop Timer14"("Count(Ticks)"=w1253) -> ("Tick Count(Ticks)"=w1254:u16)
      }
      frame #1 {
        n708 = xnode "FPGA I/O Node"("Connector1/DIO28"=w1255) -> ()  [unwired: 1 in, 1 out]
      }
      frame #2 {
        n709 = feedback-in #62(w1286) -> ()
        n710 = feedback #62(w1286) -> (w1285:u16)
        n711 = Subtract(x=w1286, y=w1285) -> (x-y=w1284:u16)
        n712 = Subtract(x=w1284, y=w1283) -> (x-y=w1259:u16)
        n713 = Number To Boolean Array(number=w1259) -> (Boolean array=w1260:bool[])
        n714 = Or Array Elements(Boolean array=w1260) -> (logical OR=w1258:bool)
        n715 = Boolean To (0,1)(Boolean="+ phase (BI D)") -> (0, 1=w1271:i16)
        n716 = Multiply(x=w1271, y="Phase count adjustment (BI D)") -> (x*y=w1268:i16)
        n717 = Boolean To (0,1)(Boolean=w1258) -> (0, 1=w1265:i16)
        n718 = To Unsigned Byte Integer(number=w1265) -> (unsigned 8bit integer=w1262:u8)
        n719 = feedback #63(i16 0) -> (w1269:i16)
        n720 = feedback #64(u8 0) -> (w1263:u8)
        n721 = Add(x=w1262, y=w1263) -> (x+y=w1261:u8)
        "Blue Late Counter (D)" <- w1261
        n722 = feedback-in #64(w1261) -> ()
        n723 = Subtract(x=w1269, y=w1268) -> (x-y=w1267:i16)
        "BI Relative phase (D)" <- w1267
        n724 = feedback-in #63(w1267) -> ()
        n725 = feedback #65(TRUE) -> (w1278:bool)
        n726 = case shown="2" "Blue Laser Operating Mode (D)" {
          tunnel: [TRUE FALSE w1292] -> w1275
          tunnel: w1278 -> [_ _ w1289]
          frame 0, Default {
          }
          frame 1 {
          }
          frame 2 {
            n727 = Not(x=w1289) -> (.not. x?=w1291:bool)
            n728 = Select(t=w1291, s="Invert BI (D)", f=w1289) -> (s? t:f=w1292:bool)
          }
        }
        n729 = Not(x=w1278) -> (.not. x?=w1274:bool)
        n730 = Select(t="Blue interlace ON count (D)", s=w1274, f="Blue interlace OFF count (D)") -> (s? t:f=w1280:u16)
        n731 = Subtract(x=w1280, y=w1259) -> (x-y=w1272:u16)
        n732 = Add(x=w1272, y=w1268) -> (x+y=w1266:u16)
        n733 = feedback-in #65(w1274) -> ()
      }
    }
  }
  n734 = while "Blue fluorescent laser interlacing (AO control direct to laser)." {
    shift-right: [w1298] -> _
    shift-left: w1 -> [w1301]
    shift-right: [w1295] -> _
    shift-left: i16 0 -> [w1293]
    stop <- FALSE stop-if-true
    n735 = flat-sequence {
      tunnel: w1301 -> [w1304]
      tunnel: [w1305] -> w1300
      tunnel: [w1304] -> w1299
      tunnel: [w1303] -> w1294
      tunnel: w1293 -> [w1303]
      tunnel: [w1308] -> w1297
      tunnel: w1300 -> [w1308]
      tunnel: [w1307] -> w1296
      tunnel: w1299 -> [w1307]
      tunnel: w1294 -> [w1306]
      tunnel: [w1318] -> w1298
      tunnel: [w1334] -> w1295
      tunnel: w1297 -> [w1346]
      tunnel: w1296 -> [w1343]
      frame #0 {
        n736 = call "Loop Timer13"("Count(Ticks)"=w1304) -> ("Tick Count(Ticks)"=w1305:u16)
      }
      frame #1 {
        n737 = xnode "FPGA I/O Node"("Connector0/AO3"=w1306) -> ()  [unwired: 1 in, 1 out]
      }
      frame #2 {
        n738 = Subtract(x="Blue OFF count (AO)", y="Blue current ON count adj (AO)") -> (x-y=w1327:u16)
        n739 = feedback-in #66(w1346) -> ()
        n740 = feedback #66(w1346) -> (w1345:u16)
        n741 = Add(x="Blue current ON count adj (AO)", y="Blue ON count (AO)") -> (x+y=w1328:u16)
        n742 = Subtract(x=w1346, y=w1345) -> (x-y=w1344:u16)
        n743 = Subtract(x=w1344, y=w1343) -> (x-y=w1311:u16)
        n744 = Number To Boolean Array(number=w1311) -> (Boolean array=w1312:bool[])
        n745 = Boolean To (0,1)(Boolean="+ phase (BI AO)") -> (0, 1=w1324:i16)
        n746 = Or Array Elements(Boolean array=w1312) -> (logical OR=w1310:bool)
        n747 = Boolean To (0,1)(Boolean=w1310) -> (0, 1=w1317:i16)
        n748 = Multiply(x=w1324, y="Phase count adjustment (BI AO)") -> (x*y=w1320:i16)
        n749 = To Unsigned Byte Integer(number=w1317) -> (unsigned 8bit integer=w1313:u8)
        n750 = feedback #67(u8 0) -> (w1315:u8)
        n751 = Add(x=w1313, y=w1315) -> (x+y=w1314:u8)
        "BI Late Counter (AO)" <- w1314
        n752 = feedback-in #67(w1314) -> ()
        n753 = feedback #68(i16 0) -> (w1321:i16)
        n754 = Subtract(x=w1321, y=w1320) -> (x-y=w1319:i16)
        "BI Relative phase (AO)" <- w1319
        n755 = feedback-in #68(w1319) -> ()
        n756 = feedback #69(TRUE) -> (w1338:bool)
        n757 = case shown="2" "BI Operating Mode (AO)" {
          tunnel: [TRUE FALSE w1362] -> w1329
          tunnel: w1338 -> [_ _ w1359]
          frame 0, Default {
          }
          frame 1 {
          }
          frame 2 {
            n758 = Not(x=w1359) -> (.not. x?=w1361:bool)
            n759 = Select(t=w1361, s="Invert BI (AO)", f=w1359) -> (s? t:f=w1362:bool)
          }
        }
        n760 = And(x=w1329, y="Blue FB On/Off") -> (x .and. y?=w1330:bool)
        n761 = case shown="True" w1330 {
          tunnel: "BI Current Out" -> [w1347 _]
          tunnel: [w1347 w1349] -> w1333
          frame False {
          }
          frame True {
            n762 = local read "Blue Intensity"() -> (w1348:i16)
            n763 = Bundle("P5"="P5", "I5"="I5", "D5"="D5") -> (w1350:cluster{"P5":i16, "I5":i16, "D5":i16})  [unwired: 1 in]
            n764 = call "Slower PID.vi"("process variable"=w1348, "reset?"="Blue FB Reset", "setpoint"="Blue FB Setpoint", "PID gains (x 2^8)"=w1350, "output range"=cluster{"output high":i16, "output low":i16} {"output high"=32767, "output low"=0} ("Green FB output range")) -> ("output"=w1349:i16)  [unwired: 10 out]
          }
        }
        n765 = Not(x=w1338) -> (.not. x?=w1335:bool)
        n766 = Select(t=w1328, s=w1335, f=w1327) -> (s? t:f=w1340:u16)
        n767 = Subtract(x=w1340, y=w1311) -> (x-y=w1322:u16)
        n768 = Add(x=w1322, y=w1320) -> (x+y=w1318:u16)
        n769 = feedback-in #69(w1335) -> ()
        n770 = Boolean To (0,1)(Boolean=w1329) -> (0, 1=w1309:i16)
        n771 = Multiply(x=w1309, y=w1333) -> (x*y=w1334:i16)
      }
    }
  }
